vi "QEditor.vi"() -> ()   [LabVIEW 2018]
uses:
  QBuilder Files/Actions_arr.ctl
  QBuilder Files/Action.ctl
  QBuilder Files/Parameters.ctl
panel:
  in  "Tab Control":enum32{"Main", "Stored Variables", "Basher"}(tab)
  in  "Actions":T1=[{"Toggle"=TRUE, "Open parameter editor"=FALSE, "Open MacroEditor"=FALSE, "Macro path"=path "", "Duration (s)"=0.001, "Parameters"=[{"Status"="ADC", "Name"="mode (0,1,2)", "Value"=0.0, "Changed"=FALSE}, {"Status"="Camera", "Name"="state (0,1)", "Value"=0.0, "Changed"=FALSE}, {"Status"="Slave", "Name"="state (0,1)", "Value"=0.0, "Changed"=FALSE}, {"Status"="Wait", "Name"="inbit (0...7)", "Value"=0.0, "Changed"=FALSE}, {"Status"="e-", "Name"="burn time (s)", "Value"=0.0, "Changed"=FALSE}, {"Status"="e-", "Name"="filament (A)", "Value"=0.0, "Changed"=FALSE}, {"Status"="e-", "Name"="enable (0,1)", "Value"=0.0, "Changed"=FALSE}, {"Status"="RW", "Name"="mode (0-13)", "Value"=0.0, "Changed"=FALSE}, {"Status"="RW", "Name"="f_start (Hz)", "Value"=0.0, "Changed"=FALSE}, {"Status"="RW", "Name"="f_stop (Hz)", "Value"=0.0, "Changed"=FALSE}, {"Status"="RW", "Name"="amplitude (V)", "Value"=0.0, "Changed"=FALSE}, {"Status"="RW", "Name"="phase dif (deg)", "Value"=0.0, "Changed"=FALSE}, {"Status"="RW", "Name"="sweep time (s)", "Value"=0.0, "Changed"=FALSE}, {"Status"="HVpuls1", "Name"="polarity (0=n)", "Value"=0.0, "Changed"=FALSE}, {"Status"="HVpuls1", "Name"="enable (0,1)", "Value"=0.0, "Changed"=FALSE}, {"Status"="HVpuls1", "Name"="amplitude (V)", "Value"=0.0, "Changed"=FALSE}, {"Status"="HVptime", "Name"="Mush on (0,1)", "Value"=0.0, "Changed"=FALSE}, {"Status"="HVptime", "Name"="Posi on (0,1)", "Value"=0.0, "Changed"=FALSE}, {"Status"="HVptime", "Name"="Cusp on (0,1)", "Value"=0.0, "Changed"=FALSE}, {"Status"="HVptime", "Name"="Posi width (s)", "Value"=0.0, "Changed"=FALSE}, {"Status"="HVptime", "Name"="Cusp delay (s)", "Value"=0.0, "Changed"=FALSE}, {"Status"="HVptime", "Name"="Cusp width (s)", "Value"=0.0, "Changed"=FALSE}, {"Status"="Dcoils", "Name"="Higaki A  (A)", "Value"=0.0, "Changed"=FALSE}, {"Status"="Dcoils", "Name"="Higaki B,C (A)", "Value"=0.0, "Changed"=FALSE}, {"Status"="Horn", "Name"="Klaxon (0,1)", "Value"=0.0, "Changed"=FALSE}, {"Status"="AMT", "Name"="posAMT (0,1)", "Value"=0.0, "Changed"=FALSE}, {"Status"="Scoop", "Name"="Acquisitions", "Value"=0.0, "Changed"=FALSE}, {"Status"="MCP", "Name"="front bias (V)", "Value"=0.0, "Changed"=FALSE}, {"Status"="MCP", "Name"="back bias (V)", "Value"=0.0, "Changed"=FALSE}, {"Status"="MCP", "Name"="phos bias (V)", "Value"=0.0, "Changed"=FALSE}, {"Status"="FI", "Name"="US bias (V)", "Value"=0.0, "Changed"=FALSE}, {"Status"="FI", "Name"="DS bias (V)", "Value"=0.0, "Changed"=FALSE}], "Comment"="", "Reps"=10}, {"Toggle"=FALSE, "Open parameter editor"=FALSE, "Open MacroEditor"=FALSE, "Macro path"=path "C:/CuspControl/Cusp/1_Macros/Antiprotons/Reservoir/v102/scoopDS__000.mac", "Duration (s)"=0.094, "Parameters"=[{"Status"="ADC", "Name"="mode (0,1,2)", "Value"=0.0, "Changed"=FALSE}, {"Status"="Camera", "Name"="state (0,1)", "Value"=0.0, "Changed"=FALSE}, {"Status"="Slave", "Name"="state (0,1)", "Value"=0.0, "Changed"=FALSE}, {"Status"="Wait", "Name"="inbit (0...7)", "Value"=0.0, "Changed"=FALSE}, {"Status"="e-", "Name"="burn time (s)", "Value"=0.0, "Changed"=FALSE}, {"Status"="e-", "Name"="filament (A)", "Value"=0.0, "Changed"=FALSE}, {"Status"="e-", "Name"="enable (0,1)", "Value"=0.0, "Changed"=FALSE}, {"Status"="RW", "Name"="mode (0-13)", "Value"=0.0, "Changed"=FALSE}, {"Status"="RW", "Name"="f_start (Hz)", "Value"=0.0, "Changed"=FALSE}, {"Status"="RW", "Name"="f_stop (Hz)", "Value"=0.0, "Changed"=FALSE}, {"Status"="RW", "Name"="amplitude (V)", "Value"=0.0, "Changed"=FALSE}, {"Status"="RW", "Name"="phase dif (deg)", "Value"=0.0, "Changed"=FALSE}, {"Status"="RW", "Name"="sweep time (s)", "Value"=0.0, "Changed"=FALSE}, {"Status"="HVpuls1", "Name"="polarity (0=n)", "Value"=0.0, "Changed"=FALSE}, {"Status"="HVpuls1", "Name"="enable (0,1)", "Value"=0.0, "Changed"=FALSE}, {"Status"="HVpuls1", "Name"="amplitude (V)", "Value"=0.0, "Changed"=FALSE}, {"Status"="HVptime", "Name"="Mush on (0,1)", "Value"=0.0, "Changed"=FALSE}, {"Status"="HVptime", "Name"="Posi on (0,1)", "Value"=0.0, "Changed"=FALSE}, {"Status"="HVptime", "Name"="Cusp on (0,1)", "Value"=0.0, "Changed"=FALSE}, {"Status"="HVptime", "Name"="Posi width (s)", "Value"=0.0, "Changed"=FALSE}, {"Status"="HVptime", "Name"="Cusp delay (s)", "Value"=0.0, "Changed"=FALSE}, {"Status"="HVptime", "Name"="Cusp width (s)", "Value"=0.0, "Changed"=FALSE}, {"Status"="Dcoils", "Name"="Higaki A  (A)", "Value"=0.0, "Changed"=FALSE}, {"Status"="Dcoils", "Name"="Higaki B,C (A)", "Value"=0.0, "Changed"=FALSE}, {"Status"="Horn", "Name"="Klaxon (0,1)", "Value"=0.0, "Changed"=FALSE}, {"Status"="AMT", "Name"="posAMT (0,1)", "Value"=0.0, "Changed"=FALSE}, {"Status"="Scoop", "Name"="Acquisitions", "Value"=0.0, "Changed"=FALSE}, {"Status"="MCP", "Name"="front bias (V)", "Value"=0.0, "Changed"=FALSE}, {"Status"="MCP", "Name"="back bias (V)", "Value"=0.0, "Changed"=FALSE}, {"Status"="MCP", "Name"="phos bias (V)", "Value"=0.0, "Changed"=FALSE}, {"Status"="FI", "Name"="US bias (V)", "Value"=0.0, "Changed"=FALSE}, {"Status"="FI", "Name"="DS bias (V)", "Value"=0.0, "Changed"=FALSE}], "Comment"="downstream dump\nno ekick", "Reps"=10}, {"Toggle"=FALSE, "Open parameter editor"=FALSE, "Open MacroEditor"=FALSE, "Macro path"=path "C:/CuspControl/Cusp/1_Macros/Antiprotons/Reservoir/v102/scoopDS__001.mac", "Duration (s)"=0.094, "Parameters"=[{"Status"="ADC", "Name"="mode (0,1,2)", "Value"=0.0, "Changed"=FALSE}, {"Status"="Camera", "Name"="state (0,1)", "Value"=0.0, "Changed"=FALSE}, {"Status"="Slave", "Name"="state (0,1)", "Value"=0.0, "Changed"=FALSE}, {"Status"="Wait", "Name"="inbit (0...7)", "Value"=0.0, "Changed"=FALSE}, {"Status"="e-", "Name"="burn time (s)", "Value"=0.0, "Changed"=FALSE}, {"Status"="e-", "Name"="filament (A)", "Value"=0.0, "Changed"=FALSE}, {"Status"="e-", "Name"="enable (0,1)", "Value"=0.0, "Changed"=FALSE}, {"Status"="RW", "Name"="mode (0-13)", "Value"=0.0, "Changed"=FALSE}, {"Status"="RW", "Name"="f_start (Hz)", "Value"=0.0, "Changed"=FALSE}, {"Status"="RW", "Name"="f_stop (Hz)", "Value"=0.0, "Changed"=FALSE}, {"Status"="RW", "Name"="amplitude (V)", "Value"=0.0, "Changed"=FALSE}, {"Status"="RW", "Name"="phase dif (deg)", "Value"=0.0, "Changed"=FALSE}, {"Status"="RW", "Name"="sweep time (s)", "Value"=0.0, "Changed"=FALSE}, {"Status"="HVpuls1", "Name"="polarity (0=n)", "Value"=0.0, "Changed"=FALSE}, {"Status"="HVpuls1", "Name"="enable (0,1)", "Value"=0.0, "Changed"=FALSE}, {"Status"="HVpuls1", "Name"="amplitude (V)", "Value"=0.0, "Changed"=FALSE}, {"Status"="HVptime", "Name"="Mush on (0,1)", "Value"=0.0, "Changed"=FALSE}, {"Status"="HVptime", "Name"="Posi on (0,1)", "Value"=0.0, "Changed"=FALSE}, {"Status"="HVptime", "Name"="Cusp on (0,1)", "Value"=0.0, "Changed"=FALSE}, {"Status"="HVptime", "Name"="Posi width (s)", "Value"=0.0, "Changed"=FALSE}, {"Status"="HVptime", "Name"="Cusp delay (s)", "Value"=0.0, "Changed"=FALSE}, {"Status"="HVptime", "Name"="Cusp width (s)", "Value"=0.0, "Changed"=FALSE}, {"Status"="Dcoils", "Name"="Higaki A  (A)", "Value"=0.0, "Changed"=FALSE}, {"Status"="Dcoils", "Name"="Higaki B,C (A)", "Value"=0.0, "Changed"=FALSE}, {"Status"="Horn", "Name"="Klaxon (0,1)", "Value"=0.0, "Changed"=FALSE}, {"Status"="AMT", "Name"="posAMT (0,1)", "Value"=0.0, "Changed"=FALSE}, {"Status"="Scoop", "Name"="Acquisitions", "Value"=0.0, "Changed"=FALSE}, {"Status"="MCP", "Name"="front bias (V)", "Value"=0.0, "Changed"=FALSE}, {"Status"="MCP", "Name"="back bias (V)", "Value"=0.0, "Changed"=FALSE}, {"Status"="MCP", "Name"="phos bias (V)", "Value"=0.0, "Changed"=FALSE}, {"Status"="FI", "Name"="US bias (V)", "Value"=0.0, "Changed"=FALSE}, {"Status"="FI", "Name"="DS bias (V)", "Value"=0.0, "Changed"=FALSE}], "Comment"="downstream dump\nno ekick", "Reps"=10}, {"Toggle"=FALSE, "Open parameter editor"=FALSE, "Open MacroEditor"=FALSE, "Macro path"=path "C:/CuspControl/Cusp/1_Macros/Antiprotons/Reservoir/v102/scoopDS__002.mac", "Duration (s)"=0.094, "Parameters"=[{"Status"="ADC", "Name"="mode (0,1,2)", "Value"=0.0, "Changed"=FALSE}, {"Status"="Camera", "Name"="state (0,1)", "Value"=0.0, "Changed"=FALSE}, {"Status"="Slave", "Name"="state (0,1)", "Value"=0.0, "Changed"=FALSE}, {"Status"="Wait", "Name"="inbit (0...7)", "Value"=0.0, "Changed"=FALSE}, {"Status"="e-", "Name"="burn time (s)", "Value"=0.0, "Changed"=FALSE}, {"Status"="e-", "Name"="filament (A)", "Value"=0.0, "Changed"=FALSE}, {"Status"="e-", "Name"="enable (0,1)", "Value"=0.0, "Changed"=FALSE}, {"Status"="RW", "Name"="mode (0-13)", "Value"=0.0, "Changed"=FALSE}, {"Status"="RW", "Name"="f_start (Hz)", "Value"=0.0, "Changed"=FALSE}, {"Status"="RW", "Name"="f_stop (Hz)", "Value"=0.0, "Changed"=FALSE}, {"Status"="RW", "Name"="amplitude (V)", "Value"=0.0, "Changed"=FALSE}, {"Status"="RW", "Name"="phase dif (deg)", "Value"=0.0, "Changed"=FALSE}, {"Status"="RW", "Name"="sweep time (s)", "Value"=0.0, "Changed"=FALSE}, {"Status"="HVpuls1", "Name"="polarity (0=n)", "Value"=0.0, "Changed"=FALSE}, {"Status"="HVpuls1", "Name"="enable (0,1)", "Value"=0.0, "Changed"=FALSE}, {"Status"="HVpuls1", "Name"="amplitude (V)", "Value"=0.0, "Changed"=FALSE}, {"Status"="HVptime", "Name"="Mush on (0,1)", "Value"=0.0, "Changed"=FALSE}, {"Status"="HVptime", "Name"="Posi on (0,1)", "Value"=0.0, "Changed"=FALSE}, {"Status"="HVptime", "Name"="Cusp on (0,1)", "Value"=0.0, "Changed"=FALSE}, {"Status"="HVptime", "Name"="Posi width (s)", "Value"=0.0, "Changed"=FALSE}, {"Status"="HVptime", "Name"="Cusp delay (s)", "Value"=0.0, "Changed"=FALSE}, {"Status"="HVptime", "Name"="Cusp width (s)", "Value"=0.0, "Changed"=FALSE}, {"Status"="Dcoils", "Name"="Higaki A  (A)", "Value"=0.0, "Changed"=FALSE}, {"Status"="Dcoils", "Name"="Higaki B,C (A)", "Value"=0.0, "Changed"=FALSE}, {"Status"="Horn", "Name"="Klaxon (0,1)", "Value"=0.0, "Changed"=FALSE}, {"Status"="AMT", "Name"="posAMT (0,1)", "Value"=0.0, "Changed"=FALSE}, {"Status"="Scoop", "Name"="Acquisitions", "Value"=0.0, "Changed"=FALSE}, {"Status"="MCP", "Name"="front bias (V)", "Value"=0.0, "Changed"=FALSE}, {"Status"="MCP", "Name"="back bias (V)", "Value"=0.0, "Changed"=FALSE}, {"Status"="MCP", "Name"="phos bias (V)", "Value"=0.0, "Changed"=FALSE}, {"Status"="FI", "Name"="US bias (V)", "Value"=0.0, "Changed"=FALSE}, {"Status"="FI", "Name"="DS bias (V)", "Value"=0.0, "Changed"=FALSE}], "Comment"="downstream dump\nno ekick", "Reps"=10}, {"Toggle"=FALSE, "Open parameter editor"=FALSE, "Open MacroEditor"=FALSE, "Macro path"=path "C:/CuspControl/Cusp/1_Macros/Antiprotons/Reservoir/v102/scoopDS__003.mac", "Duration (s)"=0.094, "Parameters"=[{"Status"="ADC", "Name"="mode (0,1,2)", "Value"=0.0, "Changed"=FALSE}, {"Status"="Camera", "Name"="state (0,1)", "Value"=0.0, "Changed"=FALSE}, {"Status"="Slave", "Name"="state (0,1)", "Value"=0.0, "Changed"=FALSE}, {"Status"="Wait", "Name"="inbit (0...7)", "Value"=0.0, "Changed"=FALSE}, {"Status"="e-", "Name"="burn time (s)", "Value"=0.0, "Changed"=FALSE}, {"Status"="e-", "Name"="filament (A)", "Value"=0.0, "Changed"=FALSE}, {"Status"="e-", "Name"="enable (0,1)", "Value"=0.0, "Changed"=FALSE}, {"Status"="RW", "Name"="mode (0-13)", "Value"=0.0, "Changed"=FALSE}, {"Status"="RW", "Name"="f_start (Hz)", "Value"=0.0, "Changed"=FALSE}, {"Status"="RW", "Name"="f_stop (Hz)", "Value"=0.0, "Changed"=FALSE}, {"Status"="RW", "Name"="amplitude (V)", "Value"=0.0, "Changed"=FALSE}, {"Status"="RW", "Name"="phase dif (deg)", "Value"=0.0, "Changed"=FALSE}, {"Status"="RW", "Name"="sweep time (s)", "Value"=0.0, "Changed"=FALSE}, {"Status"="HVpuls1", "Name"="polarity (0=n)", "Value"=0.0, "Changed"=FALSE}, {"Status"="HVpuls1", "Name"="enable (0,1)", "Value"=0.0, "Changed"=FALSE}, {"Status"="HVpuls1", "Name"="amplitude (V)", "Value"=0.0, "Changed"=FALSE}, {"Status"="HVptime", "Name"="Mush on (0,1)", "Value"=0.0, "Changed"=FALSE}, {"Status"="HVptime", "Name"="Posi on (0,1)", "Value"=0.0, "Changed"=FALSE}, {"Status"="HVptime", "Name"="Cusp on (0,1)", "Value"=0.0, "Changed"=FALSE}, {"Status"="HVptime", "Name"="Posi width (s)", "Value"=0.0, "Changed"=FALSE}, {"Status"="HVptime", "Name"="Cusp delay (s)", "Value"=0.0, "Changed"=FALSE}, {"Status"="HVptime", "Name"="Cusp width (s)", "Value"=0.0, "Changed"=FALSE}, {"Status"="Dcoils", "Name"="Higaki A  (A)", "Value"=0.0, "Changed"=FALSE}, {"Status"="Dcoils", "Name"="Higaki B,C (A)", "Value"=0.0, "Changed"=FALSE}, {"Status"="Horn", "Name"="Klaxon (0,1)", "Value"=0.0, "Changed"=FALSE}, {"Status"="AMT", "Name"="posAMT (0,1)", "Value"=0.0, "Changed"=FALSE}, {"Status"="Scoop", "Name"="Acquisitions", "Value"=0.0, "Changed"=FALSE}, {"Status"="MCP", "Name"="front bias (V)", "Value"=0.0, "Changed"=FALSE}, {"Status"="MCP", "Name"="back bias (V)", "Value"=0.0, "Changed"=FALSE}, {"Status"="MCP", "Name"="phos bias (V)", "Value"=0.0, "Changed"=FALSE}, {"Status"="FI", "Name"="US bias (V)", "Value"=0.0, "Changed"=FALSE}, {"Status"="FI", "Name"="DS bias (V)", "Value"=0.0, "Changed"=FALSE}], "Comment"="downstream dump\nno ekick", "Reps"=10}, {"Toggle"=FALSE, "Open parameter editor"=FALSE, "Open MacroEditor"=FALSE, "Macro path"=path "C:/CuspControl/Cusp/1_Macros/Antiprotons/Reservoir/v102/scoopDS__004.mac", "Duration (s)"=0.094, "Parameters"=[{"Status"="ADC", "Name"="mode (0,1,2)", "Value"=0.0, "Changed"=FALSE}, {"Status"="Camera", "Name"="state (0,1)", "Value"=0.0, "Changed"=FALSE}, {"Status"="Slave", "Name"="state (0,1)", "Value"=0.0, "Changed"=FALSE}, {"Status"="Wait", "Name"="inbit (0...7)", "Value"=0.0, "Changed"=FALSE}, {"Status"="e-", "Name"="burn time (s)", "Value"=0.0, "Changed"=FALSE}, {"Status"="e-", "Name"="filament (A)", "Value"=0.0, "Changed"=FALSE}, {"Status"="e-", "Name"="enable (0,1)", "Value"=0.0, "Changed"=FALSE}, {"Status"="RW", "Name"="mode (0-13)", "Value"=0.0, "Changed"=FALSE}, {"Status"="RW", "Name"="f_start (Hz)", "Value"=0.0, "Changed"=FALSE}, {"Status"="RW", "Name"="f_stop (Hz)", "Value"=0.0, "Changed"=FALSE}, {"Status"="RW", "Name"="amplitude (V)", "Value"=0.0, "Changed"=FALSE}, {"Status"="RW", "Name"="phase dif (deg)", "Value"=0.0, "Changed"=FALSE}, {"Status"="RW", "Name"="sweep time (s)", "Value"=0.0, "Changed"=FALSE}, {"Status"="HVpuls1", "Name"="polarity (0=n)", "Value"=0.0, "Changed"=FALSE}, {"Status"="HVpuls1", "Name"="enable (0,1)", "Value"=0.0, "Changed"=FALSE}, {"Status"="HVpuls1", "Name"="amplitude (V)", "Value"=0.0, "Changed"=FALSE}, {"Status"="HVptime", "Name"="Mush on (0,1)", "Value"=0.0, "Changed"=FALSE}, {"Status"="HVptime", "Name"="Posi on (0,1)", "Value"=0.0, "Changed"=FALSE}, {"Status"="HVptime", "Name"="Cusp on (0,1)", "Value"=0.0, "Changed"=FALSE}, {"Status"="HVptime", "Name"="Posi width (s)", "Value"=0.0, "Changed"=FALSE}, {"Status"="HVptime", "Name"="Cusp delay (s)", "Value"=0.0, "Changed"=FALSE}, {"Status"="HVptime", "Name"="Cusp width (s)", "Value"=0.0, "Changed"=FALSE}, {"Status"="Dcoils", "Name"="Higaki A  (A)", "Value"=0.0, "Changed"=FALSE}, {"Status"="Dcoils", "Name"="Higaki B,C (A)", "Value"=0.0, "Changed"=FALSE}, {"Status"="Horn", "Name"="Klaxon (0,1)", "Value"=0.0, "Changed"=FALSE}, {"Status"="AMT", "Name"="posAMT (0,1)", "Value"=0.0, "Changed"=FALSE}, {"Status"="Scoop", "Name"="Acquisitions", "Value"=0.0, "Changed"=FALSE}, {"Status"="MCP", "Name"="front bias (V)", "Value"=0.0, "Changed"=FALSE}, {"Status"="MCP", "Name"="back bias (V)", "Value"=0.0, "Changed"=FALSE}, {"Status"="MCP", "Name"="phos bias (V)", "Value"=0.0, "Changed"=FALSE}, {"Status"="FI", "Name"="US bias (V)", "Value"=0.0, "Changed"=FALSE}, {"Status"="FI", "Name"="DS bias (V)", "Value"=0.0, "Changed"=FALSE}], "Comment"="downstream dump\nno ekick", "Reps"=10}, {"Toggle"=FALSE, "Open parameter editor"=FALSE, "Open MacroEditor"=FALSE, "Macro path"=path "C:/CuspControl/Cusp/1_Macros/Antiprotons/Reservoir/v102/scoopDS__005.mac", "Duration (s)"=0.094, "Parameters"=[{"Status"="ADC", "Name"="mode (0,1,2)", "Value"=0.0, "Changed"=FALSE}, {"Status"="Camera", "Name"="state (0,1)", "Value"=0.0, "Changed"=FALSE}, {"Status"="Slave", "Name"="state (0,1)", "Value"=0.0, "Changed"=FALSE}, {"Status"="Wait", "Name"="inbit (0...7)", "Value"=0.0, "Changed"=FALSE}, {"Status"="e-", "Name"="burn time (s)", "Value"=0.0, "Changed"=FALSE}, {"Status"="e-", "Name"="filament (A)", "Value"=0.0, "Changed"=FALSE}, {"Status"="e-", "Name"="enable (0,1)", "Value"=0.0, "Changed"=FALSE}, {"Status"="RW", "Name"="mode (0-13)", "Value"=0.0, "Changed"=FALSE}, {"Status"="RW", "Name"="f_start (Hz)", "Value"=0.0, "Changed"=FALSE}, {"Status"="RW", "Name"="f_stop (Hz)", "Value"=0.0, "Changed"=FALSE}, {"Status"="RW", "Name"="amplitude (V)", "Value"=0.0, "Changed"=FALSE}, {"Status"="RW", "Name"="phase dif (deg)", "Value"=0.0, "Changed"=FALSE}, {"Status"="RW", "Name"="sweep time (s)", "Value"=0.0, "Changed"=FALSE}, {"Status"="HVpuls1", "Name"="polarity (0=n)", "Value"=0.0, "Changed"=FALSE}, {"Status"="HVpuls1", "Name"="enable (0,1)", "Value"=0.0, "Changed"=FALSE}, {"Status"="HVpuls1", "Name"="amplitude (V)", "Value"=0.0, "Changed"=FALSE}, {"Status"="HVptime", "Name"="Mush on (0,1)", "Value"=0.0, "Changed"=FALSE}, {"Status"="HVptime", "Name"="Posi on (0,1)", "Value"=0.0, "Changed"=FALSE}, {"Status"="HVptime", "Name"="Cusp on (0,1)", "Value"=0.0, "Changed"=FALSE}, {"Status"="HVptime", "Name"="Posi width (s)", "Value"=0.0, "Changed"=FALSE}, {"Status"="HVptime", "Name"="Cusp delay (s)", "Value"=0.0, "Changed"=FALSE}, {"Status"="HVptime", "Name"="Cusp width (s)", "Value"=0.0, "Changed"=FALSE}, {"Status"="Dcoils", "Name"="Higaki A  (A)", "Value"=0.0, "Changed"=FALSE}, {"Status"="Dcoils", "Name"="Higaki B,C (A)", "Value"=0.0, "Changed"=FALSE}, {"Status"="Horn", "Name"="Klaxon (0,1)", "Value"=0.0, "Changed"=FALSE}, {"Status"="AMT", "Name"="posAMT (0,1)", "Value"=0.0, "Changed"=FALSE}, {"Status"="Scoop", "Name"="Acquisitions", "Value"=0.0, "Changed"=FALSE}, {"Status"="MCP", "Name"="front bias (V)", "Value"=0.0, "Changed"=FALSE}, {"Status"="MCP", "Name"="back bias (V)", "Value"=0.0, "Changed"=FALSE}, {"Status"="MCP", "Name"="phos bias (V)", "Value"=0.0, "Changed"=FALSE}, {"Status"="FI", "Name"="US bias (V)", "Value"=0.0, "Changed"=FALSE}, {"Status"="FI", "Name"="DS bias (V)", "Value"=0.0, "Changed"=FALSE}], "Comment"="downstream dump\nno ekick", "Reps"=10}, {"Toggle"=FALSE, "Open parameter editor"=FALSE, "Open MacroEditor"=FALSE, "Macro path"=path "C:/CuspControl/Cusp/1_Macros/Antiprotons/Reservoir/v102/scoopDS__006.mac", "Duration (s)"=0.094, "Parameters"=[{"Status"="ADC", "Name"="mode (0,1,2)", "Value"=0.0, "Changed"=FALSE}, {"Status"="Camera", "Name"="state (0,1)", "Value"=0.0, "Changed"=FALSE}, {"Status"="Slave", "Name"="state (0,1)", "Value"=0.0, "Changed"=FALSE}, {"Status"="Wait", "Name"="inbit (0...7)", "Value"=0.0, "Changed"=FALSE}, {"Status"="e-", "Name"="burn time (s)", "Value"=0.0, "Changed"=FALSE}, {"Status"="e-", "Name"="filament (A)", "Value"=0.0, "Changed"=FALSE}, {"Status"="e-", "Name"="enable (0,1)", "Value"=0.0, "Changed"=FALSE}, {"Status"="RW", "Name"="mode (0-13)", "Value"=0.0, "Changed"=FALSE}, {"Status"="RW", "Name"="f_start (Hz)", "Value"=0.0, "Changed"=FALSE}, {"Status"="RW", "Name"="f_stop (Hz)", "Value"=0.0, "Changed"=FALSE}, {"Status"="RW", "Name"="amplitude (V)", "Value"=0.0, "Changed"=FALSE}, {"Status"="RW", "Name"="phase dif (deg)", "Value"=0.0, "Changed"=FALSE}, {"Status"="RW", "Name"="sweep time (s)", "Value"=0.0, "Changed"=FALSE}, {"Status"="HVpuls1", "Name"="polarity (0=n)", "Value"=0.0, "Changed"=FALSE}, {"Status"="HVpuls1", "Name"="enable (0,1)", "Value"=0.0, "Changed"=FALSE}, {"Status"="HVpuls1", "Name"="amplitude (V)", "Value"=0.0, "Changed"=FALSE}, {"Status"="HVptime", "Name"="Mush on (0,1)", "Value"=0.0, "Changed"=FALSE}, {"Status"="HVptime", "Name"="Posi on (0,1)", "Value"=0.0, "Changed"=FALSE}, {"Status"="HVptime", "Name"="Cusp on (0,1)", "Value"=0.0, "Changed"=FALSE}, {"Status"="HVptime", "Name"="Posi width (s)", "Value"=0.0, "Changed"=FALSE}, {"Status"="HVptime", "Name"="Cusp delay (s)", "Value"=0.0, "Changed"=FALSE}, {"Status"="HVptime", "Name"="Cusp width (s)", "Value"=0.0, "Changed"=FALSE}, {"Status"="Dcoils", "Name"="Higaki A  (A)", "Value"=0.0, "Changed"=FALSE}, {"Status"="Dcoils", "Name"="Higaki B,C (A)", "Value"=0.0, "Changed"=FALSE}, {"Status"="Horn", "Name"="Klaxon (0,1)", "Value"=0.0, "Changed"=FALSE}, {"Status"="AMT", "Name"="posAMT (0,1)", "Value"=0.0, "Changed"=FALSE}, {"Status"="Scoop", "Name"="Acquisitions", "Value"=0.0, "Changed"=FALSE}, {"Status"="MCP", "Name"="front bias (V)", "Value"=0.0, "Changed"=FALSE}, {"Status"="MCP", "Name"="back bias (V)", "Value"=0.0, "Changed"=FALSE}, {"Status"="MCP", "Name"="phos bias (V)", "Value"=0.0, "Changed"=FALSE}, {"Status"="FI", "Name"="US bias (V)", "Value"=0.0, "Changed"=FALSE}, {"Status"="FI", "Name"="DS bias (V)", "Value"=0.0, "Changed"=FALSE}], "Comment"="downstream dump\nno ekick", "Reps"=10}, {"Toggle"=FALSE, "Open parameter editor"=FALSE, "Open MacroEditor"=FALSE, "Macro path"=path "C:/CuspControl/Cusp/1_Macros/Antiprotons/Reservoir/v102/scoopDS__007.mac", "Duration (s)"=0.094, "Parameters"=[{"Status"="ADC", "Name"="mode (0,1,2)", "Value"=0.0, "Changed"=FALSE}, {"Status"="Camera", "Name"="state (0,1)", "Value"=0.0, "Changed"=FALSE}, {"Status"="Slave", "Name"="state (0,1)", "Value"=0.0, "Changed"=FALSE}, {"Status"="Wait", "Name"="inbit (0...7)", "Value"=0.0, "Changed"=FALSE}, {"Status"="e-", "Name"="burn time (s)", "Value"=0.0, "Changed"=FALSE}, {"Status"="e-", "Name"="filament (A)", "Value"=0.0, "Changed"=FALSE}, {"Status"="e-", "Name"="enable (0,1)", "Value"=0.0, "Changed"=FALSE}, {"Status"="RW", "Name"="mode (0-13)", "Value"=0.0, "Changed"=FALSE}, {"Status"="RW", "Name"="f_start (Hz)", "Value"=0.0, "Changed"=FALSE}, {"Status"="RW", "Name"="f_stop (Hz)", "Value"=0.0, "Changed"=FALSE}, {"Status"="RW", "Name"="amplitude (V)", "Value"=0.0, "Changed"=FALSE}, {"Status"="RW", "Name"="phase dif (deg)", "Value"=0.0, "Changed"=FALSE}, {"Status"="RW", "Name"="sweep time (s)", "Value"=0.0, "Changed"=FALSE}, {"Status"="HVpuls1", "Name"="polarity (0=n)", "Value"=0.0, "Changed"=FALSE}, {"Status"="HVpuls1", "Name"="enable (0,1)", "Value"=0.0, "Changed"=FALSE}, {"Status"="HVpuls1", "Name"="amplitude (V)", "Value"=0.0, "Changed"=FALSE}, {"Status"="HVptime", "Name"="Mush on (0,1)", "Value"=0.0, "Changed"=FALSE}, {"Status"="HVptime", "Name"="Posi on (0,1)", "Value"=0.0, "Changed"=FALSE}, {"Status"="HVptime", "Name"="Cusp on (0,1)", "Value"=0.0, "Changed"=FALSE}, {"Status"="HVptime", "Name"="Posi width (s)", "Value"=0.0, "Changed"=FALSE}, {"Status"="HVptime", "Name"="Cusp delay (s)", "Value"=0.0, "Changed"=FALSE}, {"Status"="HVptime", "Name"="Cusp width (s)", "Value"=0.0, "Changed"=FALSE}, {"Status"="Dcoils", "Name"="Higaki A  (A)", "Value"=0.0, "Changed"=FALSE}, {"Status"="Dcoils", "Name"="Higaki B,C (A)", "Value"=0.0, "Changed"=FALSE}, {"Status"="Horn", "Name"="Klaxon (0,1)", "Value"=0.0, "Changed"=FALSE}, {"Status"="AMT", "Name"="posAMT (0,1)", "Value"=0.0, "Changed"=FALSE}, {"Status"="Scoop", "Name"="Acquisitions", "Value"=0.0, "Changed"=FALSE}, {"Status"="MCP", "Name"="front bias (V)", "Value"=0.0, "Changed"=FALSE}, {"Status"="MCP", "Name"="back bias (V)", "Value"=0.0, "Changed"=FALSE}, {"Status"="MCP", "Name"="phos bias (V)", "Value"=0.0, "Changed"=FALSE}, {"Status"="FI", "Name"="US bias (V)", "Value"=0.0, "Changed"=FALSE}, {"Status"="FI", "Name"="DS bias (V)", "Value"=0.0, "Changed"=FALSE}], "Comment"="downstream dump\nno ekick", "Reps"=10}, {"Toggle"=FALSE, "Open parameter editor"=FALSE, "Open MacroEditor"=FALSE, "Macro path"=path "C:/CuspControl/Cusp/1_Macros/Antiprotons/Reservoir/v102/scoopDS__008.mac", "Duration (s)"=0.094, "Parameters"=[{"Status"="ADC", "Name"="mode (0,1,2)", "Value"=0.0, "Changed"=FALSE}, {"Status"="Camera", "Name"="state (0,1)", "Value"=0.0, "Changed"=FALSE}, {"Status"="Slave", "Name"="state (0,1)", "Value"=0.0, "Changed"=FALSE}, {"Status"="Wait", "Name"="inbit (0...7)", "Value"=0.0, "Changed"=FALSE}, {"Status"="e-", "Name"="burn time (s)", "Value"=0.0, "Changed"=FALSE}, {"Status"="e-", "Name"="filament (A)", "Value"=0.0, "Changed"=FALSE}, {"Status"="e-", "Name"="enable (0,1)", "Value"=0.0, "Changed"=FALSE}, {"Status"="RW", "Name"="mode (0-13)", "Value"=0.0, "Changed"=FALSE}, {"Status"="RW", "Name"="f_start (Hz)", "Value"=0.0, "Changed"=FALSE}, {"Status"="RW", "Name"="f_stop (Hz)", "Value"=0.0, "Changed"=FALSE}, {"Status"="RW", "Name"="amplitude (V)", "Value"=0.0, "Changed"=FALSE}, {"Status"="RW", "Name"="phase dif (deg)", "Value"=0.0, "Changed"=FALSE}, {"Status"="RW", "Name"="sweep time (s)", "Value"=0.0, "Changed"=FALSE}, {"Status"="HVpuls1", "Name"="polarity (0=n)", "Value"=0.0, "Changed"=FALSE}, {"Status"="HVpuls1", "Name"="enable (0,1)", "Value"=0.0, "Changed"=FALSE}, {"Status"="HVpuls1", "Name"="amplitude (V)", "Value"=0.0, "Changed"=FALSE}, {"Status"="HVptime", "Name"="Mush on (0,1)", "Value"=0.0, "Changed"=FALSE}, {"Status"="HVptime", "Name"="Posi on (0,1)", "Value"=0.0, "Changed"=FALSE}, {"Status"="HVptime", "Name"="Cusp on (0,1)", "Value"=0.0, "Changed"=FALSE}, {"Status"="HVptime", "Name"="Posi width (s)", "Value"=0.0, "Changed"=FALSE}, {"Status"="HVptime", "Name"="Cusp delay (s)", "Value"=0.0, "Changed"=FALSE}, {"Status"="HVptime", "Name"="Cusp width (s)", "Value"=0.0, "Changed"=FALSE}, {"Status"="Dcoils", "Name"="Higaki A  (A)", "Value"=0.0, "Changed"=FALSE}, {"Status"="Dcoils", "Name"="Higaki B,C (A)", "Value"=0.0, "Changed"=FALSE}, {"Status"="Horn", "Name"="Klaxon (0,1)", "Value"=0.0, "Changed"=FALSE}, {"Status"="AMT", "Name"="posAMT (0,1)", "Value"=0.0, "Changed"=FALSE}, {"Status"="Scoop", "Name"="Acquisitions", "Value"=0.0, "Changed"=FALSE}, {"Status"="MCP", "Name"="front bias (V)", "Value"=0.0, "Changed"=FALSE}, {"Status"="MCP", "Name"="back bias (V)", "Value"=0.0, "Changed"=FALSE}, {"Status"="MCP", "Name"="phos bias (V)", "Value"=0.0, "Changed"=FALSE}, {"Status"="FI", "Name"="US bias (V)", "Value"=0.0, "Changed"=FALSE}, {"Status"="FI", "Name"="DS bias (V)", "Value"=0.0, "Changed"=FALSE}], "Comment"="downstream dump\nno ekick", "Reps"=10}, {"Toggle"=FALSE, "Open parameter editor"=FALSE, "Open MacroEditor"=FALSE, "Macro path"=path "C:/CuspControl/Cusp/1_Macros/Antiprotons/Reservoir/v102/scoopDS__009.mac", "Duration (s)"=0.094, "Parameters"=[{"Status"="ADC", "Name"="mode (0,1,2)", "Value"=0.0, "Changed"=FALSE}, {"Status"="Camera", "Name"="state (0,1)", "Value"=0.0, "Changed"=FALSE}, {"Status"="Slave", "Name"="state (0,1)", "Value"=0.0, "Changed"=FALSE}, {"Status"="Wait", "Name"="inbit (0...7)", "Value"=0.0, "Changed"=FALSE}, {"Status"="e-", "Name"="burn time (s)", "Value"=0.0, "Changed"=FALSE}, {"Status"="e-", "Name"="filament (A)", "Value"=0.0, "Changed"=FALSE}, {"Status"="e-", "Name"="enable (0,1)", "Value"=0.0, "Changed"=FALSE}, {"Status"="RW", "Name"="mode (0-13)", "Value"=0.0, "Changed"=FALSE}, {"Status"="RW", "Name"="f_start (Hz)", "Value"=0.0, "Changed"=FALSE}, {"Status"="RW", "Name"="f_stop (Hz)", "Value"=0.0, "Changed"=FALSE}, {"Status"="RW", "Name"="amplitude (V)", "Value"=0.0, "Changed"=FALSE}, {"Status"="RW", "Name"="phase dif (deg)", "Value"=0.0, "Changed"=FALSE}, {"Status"="RW", "Name"="sweep time (s)", "Value"=0.0, "Changed"=FALSE}, {"Status"="HVpuls1", "Name"="polarity (0=n)", "Value"=0.0, "Changed"=FALSE}, {"Status"="HVpuls1", "Name"="enable (0,1)", "Value"=0.0, "Changed"=FALSE}, {"Status"="HVpuls1", "Name"="amplitude (V)", "Value"=0.0, "Changed"=FALSE}, {"Status"="HVptime", "Name"="Mush on (0,1)", "Value"=0.0, "Changed"=FALSE}, {"Status"="HVptime", "Name"="Posi on (0,1)", "Value"=0.0, "Changed"=FALSE}, {"Status"="HVptime", "Name"="Cusp on (0,1)", "Value"=0.0, "Changed"=FALSE}, {"Status"="HVptime", "Name"="Posi width (s)", "Value"=0.0, "Changed"=FALSE}, {"Status"="HVptime", "Name"="Cusp delay (s)", "Value"=0.0, "Changed"=FALSE}, {"Status"="HVptime", "Name"="Cusp width (s)", "Value"=0.0, "Changed"=FALSE}, {"Status"="Dcoils", "Name"="Higaki A  (A)", "Value"=0.0, "Changed"=FALSE}, {"Status"="Dcoils", "Name"="Higaki B,C (A)", "Value"=0.0, "Changed"=FALSE}, {"Status"="Horn", "Name"="Klaxon (0,1)", "Value"=0.0, "Changed"=FALSE}, {"Status"="AMT", "Name"="posAMT (0,1)", "Value"=0.0, "Changed"=FALSE}, {"Status"="Scoop", "Name"="Acquisitions", "Value"=0.0, "Changed"=FALSE}, {"Status"="MCP", "Name"="front bias (V)", "Value"=0.0, "Changed"=FALSE}, {"Status"="MCP", "Name"="back bias (V)", "Value"=0.0, "Changed"=FALSE}, {"Status"="MCP", "Name"="phos bias (V)", "Value"=0.0, "Changed"=FALSE}, {"Status"="FI", "Name"="US bias (V)", "Value"=0.0, "Changed"=FALSE}, {"Status"="FI", "Name"="DS bias (V)", "Value"=0.0, "Changed"=FALSE}], "Comment"="downstream dump\nno ekick", "Reps"=10}, {"Toggle"=FALSE, "Open parameter editor"=FALSE, "Open MacroEditor"=FALSE, "Macro path"=path "C:/CuspControl/Cusp/1_Macros/Antiprotons/Reservoir/v102/scoopDS__010.mac", "Duration (s)"=0.094, "Parameters"=[{"Status"="ADC", "Name"="mode (0,1,2)", "Value"=0.0, "Changed"=FALSE}, {"Status"="Camera", "Name"="state (0,1)", "Value"=0.0, "Changed"=FALSE}, {"Status"="Slave", "Name"="state (0,1)", "Value"=0.0, "Changed"=FALSE}, {"Status"="Wait", "Name"="inbit (0...7)", "Value"=0.0, "Changed"=FALSE}, {"Status"="e-", "Name"="burn time (s)", "Value"=0.0, "Changed"=FALSE}, {"Status"="e-", "Name"="filament (A)", "Value"=0.0, "Changed"=FALSE}, {"Status"="e-", "Name"="enable (0,1)", "Value"=0.0, "Changed"=FALSE}, {"Status"="RW", "Name"="mode (0-13)", "Value"=0.0, "Changed"=FALSE}, {"Status"="RW", "Name"="f_start (Hz)", "Value"=0.0, "Changed"=FALSE}, {"Status"="RW", "Name"="f_stop (Hz)", "Value"=0.0, "Changed"=FALSE}, {"Status"="RW", "Name"="amplitude (V)", "Value"=0.0, "Changed"=FALSE}, {"Status"="RW", "Name"="phase dif (deg)", "Value"=0.0, "Changed"=FALSE}, {"Status"="RW", "Name"="sweep time (s)", "Value"=0.0, "Changed"=FALSE}, {"Status"="HVpuls1", "Name"="polarity (0=n)", "Value"=0.0, "Changed"=FALSE}, {"Status"="HVpuls1", "Name"="enable (0,1)", "Value"=0.0, "Changed"=FALSE}, {"Status"="HVpuls1", "Name"="amplitude (V)", "Value"=0.0, "Changed"=FALSE}, {"Status"="HVptime", "Name"="Mush on (0,1)", "Value"=0.0, "Changed"=FALSE}, {"Status"="HVptime", "Name"="Posi on (0,1)", "Value"=0.0, "Changed"=FALSE}, {"Status"="HVptime", "Name"="Cusp on (0,1)", "Value"=0.0, "Changed"=FALSE}, {"Status"="HVptime", "Name"="Posi width (s)", "Value"=0.0, "Changed"=FALSE}, {"Status"="HVptime", "Name"="Cusp delay (s)", "Value"=0.0, "Changed"=FALSE}, {"Status"="HVptime", "Name"="Cusp width (s)", "Value"=0.0, "Changed"=FALSE}, {"Status"="Dcoils", "Name"="Higaki A  (A)", "Value"=0.0, "Changed"=FALSE}, {"Status"="Dcoils", "Name"="Higaki B,C (A)", "Value"=0.0, "Changed"=FALSE}, {"Status"="Horn", "Name"="Klaxon (0,1)", "Value"=0.0, "Changed"=FALSE}, {"Status"="AMT", "Name"="posAMT (0,1)", "Value"=0.0, "Changed"=FALSE}, {"Status"="Scoop", "Name"="Acquisitions", "Value"=0.0, "Changed"=FALSE}, {"Status"="MCP", "Name"="front bias (V)", "Value"=0.0, "Changed"=FALSE}, {"Status"="MCP", "Name"="back bias (V)", "Value"=0.0, "Changed"=FALSE}, {"Status"="MCP", "Name"="phos bias (V)", "Value"=0.0, "Changed"=FALSE}, {"Status"="FI", "Name"="US bias (V)", "Value"=0.0, "Changed"=FALSE}, {"Status"="FI", "Name"="DS bias (V)", "Value"=0.0, "Changed"=FALSE}], "Comment"="downstream dump\nno ekick", "Reps"=10}, {"Toggle"=FALSE, "Open parameter editor"=FALSE, "Open MacroEditor"=FALSE, "Macro path"=path "C:/CuspControl/Cusp/1_Macros/Antiprotons/Reservoir/v102/scoopDS__011.mac", "Duration (s)"=0.094, "Parameters"=[{"Status"="ADC", "Name"="mode (0,1,2)", "Value"=0.0, "Changed"=FALSE}, {"Status"="Camera", "Name"="state (0,1)", "Value"=0.0, "Changed"=FALSE}, {"Status"="Slave", "Name"="state (0,1)", "Value"=0.0, "Changed"=FALSE}, {"Status"="Wait", "Name"="inbit (0...7)", "Value"=0.0, "Changed"=FALSE}, {"Status"="e-", "Name"="burn time (s)", "Value"=0.0, "Changed"=FALSE}, {"Status"="e-", "Name"="filament (A)", "Value"=0.0, "Changed"=FALSE}, {"Status"="e-", "Name"="enable (0,1)", "Value"=0.0, "Changed"=FALSE}, {"Status"="RW", "Name"="mode (0-13)", "Value"=0.0, "Changed"=FALSE}, {"Status"="RW", "Name"="f_start (Hz)", "Value"=0.0, "Changed"=FALSE}, {"Status"="RW", "Name"="f_stop (Hz)", "Value"=0.0, "Changed"=FALSE}, {"Status"="RW", "Name"="amplitude (V)", "Value"=0.0, "Changed"=FALSE}, {"Status"="RW", "Name"="phase dif (deg)", "Value"=0.0, "Changed"=FALSE}, {"Status"="RW", "Name"="sweep time (s)", "Value"=0.0, "Changed"=FALSE}, {"Status"="HVpuls1", "Name"="polarity (0=n)", "Value"=0.0, "Changed"=FALSE}, {"Status"="HVpuls1", "Name"="enable (0,1)", "Value"=0.0, "Changed"=FALSE}, {"Status"="HVpuls1", "Name"="amplitude (V)", "Value"=0.0, "Changed"=FALSE}, {"Status"="HVptime", "Name"="Mush on (0,1)", "Value"=0.0, "Changed"=FALSE}, {"Status"="HVptime", "Name"="Posi on (0,1)", "Value"=0.0, "Changed"=FALSE}, {"Status"="HVptime", "Name"="Cusp on (0,1)", "Value"=0.0, "Changed"=FALSE}, {"Status"="HVptime", "Name"="Posi width (s)", "Value"=0.0, "Changed"=FALSE}, {"Status"="HVptime", "Name"="Cusp delay (s)", "Value"=0.0, "Changed"=FALSE}, {"Status"="HVptime", "Name"="Cusp width (s)", "Value"=0.0, "Changed"=FALSE}, {"Status"="Dcoils", "Name"="Higaki A  (A)", "Value"=0.0, "Changed"=FALSE}, {"Status"="Dcoils", "Name"="Higaki B,C (A)", "Value"=0.0, "Changed"=FALSE}, {"Status"="Horn", "Name"="Klaxon (0,1)", "Value"=0.0, "Changed"=FALSE}, {"Status"="AMT", "Name"="posAMT (0,1)", "Value"=0.0, "Changed"=FALSE}, {"Status"="Scoop", "Name"="Acquisitions", "Value"=0.0, "Changed"=FALSE}, {"Status"="MCP", "Name"="front bias (V)", "Value"=0.0, "Changed"=FALSE}, {"Status"="MCP", "Name"="back bias (V)", "Value"=0.0, "Changed"=FALSE}, {"Status"="MCP", "Name"="phos bias (V)", "Value"=0.0, "Changed"=FALSE}, {"Status"="FI", "Name"="US bias (V)", "Value"=0.0, "Changed"=FALSE}, {"Status"="FI", "Name"="DS bias (V)", "Value"=0.0, "Changed"=FALSE}], "Comment"="downstream dump\nno ekick", "Reps"=10}, {"Toggle"=FALSE, "Open parameter editor"=FALSE, "Open MacroEditor"=FALSE, "Macro path"=path "C:/CuspControl/Cusp/1_Macros/Antiprotons/Reservoir/v102/scoopDS__012.mac", "Duration (s)"=0.094, "Parameters"=[{"Status"="ADC", "Name"="mode (0,1,2)", "Value"=0.0, "Changed"=FALSE}, {"Status"="Camera", "Name"="state (0,1)", "Value"=0.0, "Changed"=FALSE}, {"Status"="Slave", "Name"="state (0,1)", "Value"=0.0, "Changed"=FALSE}, {"Status"="Wait", "Name"="inbit (0...7)", "Value"=0.0, "Changed"=FALSE}, {"Status"="e-", "Name"="burn time (s)", "Value"=0.0, "Changed"=FALSE}, {"Status"="e-", "Name"="filament (A)", "Value"=0.0, "Changed"=FALSE}, {"Status"="e-", "Name"="enable (0,1)", "Value"=0.0, "Changed"=FALSE}, {"Status"="RW", "Name"="mode (0-13)", "Value"=0.0, "Changed"=FALSE}, {"Status"="RW", "Name"="f_start (Hz)", "Value"=0.0, "Changed"=FALSE}, {"Status"="RW", "Name"="f_stop (Hz)", "Value"=0.0, "Changed"=FALSE}, {"Status"="RW", "Name"="amplitude (V)", "Value"=0.0, "Changed"=FALSE}, {"Status"="RW", "Name"="phase dif (deg)", "Value"=0.0, "Changed"=FALSE}, {"Status"="RW", "Name"="sweep time (s)", "Value"=0.0, "Changed"=FALSE}, {"Status"="HVpuls1", "Name"="polarity (0=n)", "Value"=0.0, "Changed"=FALSE}, {"Status"="HVpuls1", "Name"="enable (0,1)", "Value"=0.0, "Changed"=FALSE}, {"Status"="HVpuls1", "Name"="amplitude (V)", "Value"=0.0, "Changed"=FALSE}, {"Status"="HVptime", "Name"="Mush on (0,1)", "Value"=0.0, "Changed"=FALSE}, {"Status"="HVptime", "Name"="Posi on (0,1)", "Value"=0.0, "Changed"=FALSE}, {"Status"="HVptime", "Name"="Cusp on (0,1)", "Value"=0.0, "Changed"=FALSE}, {"Status"="HVptime", "Name"="Posi width (s)", "Value"=0.0, "Changed"=FALSE}, {"Status"="HVptime", "Name"="Cusp delay (s)", "Value"=0.0, "Changed"=FALSE}, {"Status"="HVptime", "Name"="Cusp width (s)", "Value"=0.0, "Changed"=FALSE}, {"Status"="Dcoils", "Name"="Higaki A  (A)", "Value"=0.0, "Changed"=FALSE}, {"Status"="Dcoils", "Name"="Higaki B,C (A)", "Value"=0.0, "Changed"=FALSE}, {"Status"="Horn", "Name"="Klaxon (0,1)", "Value"=0.0, "Changed"=FALSE}, {"Status"="AMT", "Name"="posAMT (0,1)", "Value"=0.0, "Changed"=FALSE}, {"Status"="Scoop", "Name"="Acquisitions", "Value"=0.0, "Changed"=FALSE}, {"Status"="MCP", "Name"="front bias (V)", "Value"=0.0, "Changed"=FALSE}, {"Status"="MCP", "Name"="back bias (V)", "Value"=0.0, "Changed"=FALSE}, {"Status"="MCP", "Name"="phos bias (V)", "Value"=0.0, "Changed"=FALSE}, {"Status"="FI", "Name"="US bias (V)", "Value"=0.0, "Changed"=FALSE}, {"Status"="FI", "Name"="DS bias (V)", "Value"=0.0, "Changed"=FALSE}], "Comment"="downstream dump\nno ekick", "Reps"=10}, {"Toggle"=FALSE, "Open parameter editor"=FALSE, "Open MacroEditor"=FALSE, "Macro path"=path "C:/CuspControl/Cusp/1_Macros/Antiprotons/Reservoir/v102/scoopDS__013.mac", "Duration (s)"=0.094, "Parameters"=[{"Status"="ADC", "Name"="mode (0,1,2)", "Value"=0.0, "Changed"=FALSE}, {"Status"="Camera", "Name"="state (0,1)", "Value"=0.0, "Changed"=FALSE}, {"Status"="Slave", "Name"="state (0,1)", "Value"=0.0, "Changed"=FALSE}, {"Status"="Wait", "Name"="inbit (0...7)", "Value"=0.0, "Changed"=FALSE}, {"Status"="e-", "Name"="burn time (s)", "Value"=0.0, "Changed"=FALSE}, {"Status"="e-", "Name"="filament (A)", "Value"=0.0, "Changed"=FALSE}, {"Status"="e-", "Name"="enable (0,1)", "Value"=0.0, "Changed"=FALSE}, {"Status"="RW", "Name"="mode (0-13)", "Value"=0.0, "Changed"=FALSE}, {"Status"="RW", "Name"="f_start (Hz)", "Value"=0.0, "Changed"=FALSE}, {"Status"="RW", "Name"="f_stop (Hz)", "Value"=0.0, "Changed"=FALSE}, {"Status"="RW", "Name"="amplitude (V)", "Value"=0.0, "Changed"=FALSE}, {"Status"="RW", "Name"="phase dif (deg)", "Value"=0.0, "Changed"=FALSE}, {"Status"="RW", "Name"="sweep time (s)", "Value"=0.0, "Changed"=FALSE}, {"Status"="HVpuls1", "Name"="polarity (0=n)", "Value"=0.0, "Changed"=FALSE}, {"Status"="HVpuls1", "Name"="enable (0,1)", "Value"=0.0, "Changed"=FALSE}, {"Status"="HVpuls1", "Name"="amplitude (V)", "Value"=0.0, "Changed"=FALSE}, {"Status"="HVptime", "Name"="Mush on (0,1)", "Value"=0.0, "Changed"=FALSE}, {"Status"="HVptime", "Name"="Posi on (0,1)", "Value"=0.0, "Changed"=FALSE}, {"Status"="HVptime", "Name"="Cusp on (0,1)", "Value"=0.0, "Changed"=FALSE}, {"Status"="HVptime", "Name"="Posi width (s)", "Value"=0.0, "Changed"=FALSE}, {"Status"="HVptime", "Name"="Cusp delay (s)", "Value"=0.0, "Changed"=FALSE}, {"Status"="HVptime", "Name"="Cusp width (s)", "Value"=0.0, "Changed"=FALSE}, {"Status"="Dcoils", "Name"="Higaki A  (A)", "Value"=0.0, "Changed"=FALSE}, {"Status"="Dcoils", "Name"="Higaki B,C (A)", "Value"=0.0, "Changed"=FALSE}, {"Status"="Horn", "Name"="Klaxon (0,1)", "Value"=0.0, "Changed"=FALSE}, {"Status"="AMT", "Name"="posAMT (0,1)", "Value"=0.0, "Changed"=FALSE}, {"Status"="Scoop", "Name"="Acquisitions", "Value"=0.0, "Changed"=FALSE}, {"Status"="MCP", "Name"="front bias (V)", "Value"=0.0, "Changed"=FALSE}, {"Status"="MCP", "Name"="back bias (V)", "Value"=0.0, "Changed"=FALSE}, {"Status"="MCP", "Name"="phos bias (V)", "Value"=0.0, "Changed"=FALSE}, {"Status"="FI", "Name"="US bias (V)", "Value"=0.0, "Changed"=FALSE}, {"Status"="FI", "Name"="DS bias (V)", "Value"=0.0, "Changed"=FALSE}], "Comment"="downstream dump\nno ekick", "Reps"=10}, {"Toggle"=FALSE, "Open parameter editor"=FALSE, "Open MacroEditor"=FALSE, "Macro path"=path "C:/CuspControl/Cusp/1_Macros/Antiprotons/Reservoir/v102/scoopDS__014.mac", "Duration (s)"=0.094, "Parameters"=[{"Status"="ADC", "Name"="mode (0,1,2)", "Value"=0.0, "Changed"=FALSE}, {"Status"="Camera", "Name"="state (0,1)", "Value"=0.0, "Changed"=FALSE}, {"Status"="Slave", "Name"="state (0,1)", "Value"=0.0, "Changed"=FALSE}, {"Status"="Wait", "Name"="inbit (0...7)", "Value"=0.0, "Changed"=FALSE}, {"Status"="e-", "Name"="burn time (s)", "Value"=0.0, "Changed"=FALSE}, {"Status"="e-", "Name"="filament (A)", "Value"=0.0, "Changed"=FALSE}, {"Status"="e-", "Name"="enable (0,1)", "Value"=0.0, "Changed"=FALSE}, {"Status"="RW", "Name"="mode (0-13)", "Value"=0.0, "Changed"=FALSE}, {"Status"="RW", "Name"="f_start (Hz)", "Value"=0.0, "Changed"=FALSE}, {"Status"="RW", "Name"="f_stop (Hz)", "Value"=0.0, "Changed"=FALSE}, {"Status"="RW", "Name"="amplitude (V)", "Value"=0.0, "Changed"=FALSE}, {"Status"="RW", "Name"="phase dif (deg)", "Value"=0.0, "Changed"=FALSE}, {"Status"="RW", "Name"="sweep time (s)", "Value"=0.0, "Changed"=FALSE}, {"Status"="HVpuls1", "Name"="polarity (0=n)", "Value"=0.0, "Changed"=FALSE}, {"Status"="HVpuls1", "Name"="enable (0,1)", "Value"=0.0, "Changed"=FALSE}, {"Status"="HVpuls1", "Name"="amplitude (V)", "Value"=0.0, "Changed"=FALSE}, {"Status"="HVptime", "Name"="Mush on (0,1)", "Value"=0.0, "Changed"=FALSE}, {"Status"="HVptime", "Name"="Posi on (0,1)", "Value"=0.0, "Changed"=FALSE}, {"Status"="HVptime", "Name"="Cusp on (0,1)", "Value"=0.0, "Changed"=FALSE}, {"Status"="HVptime", "Name"="Posi width (s)", "Value"=0.0, "Changed"=FALSE}, {"Status"="HVptime", "Name"="Cusp delay (s)", "Value"=0.0, "Changed"=FALSE}, {"Status"="HVptime", "Name"="Cusp width (s)", "Value"=0.0, "Changed"=FALSE}, {"Status"="Dcoils", "Name"="Higaki A  (A)", "Value"=0.0, "Changed"=FALSE}, {"Status"="Dcoils", "Name"="Higaki B,C (A)", "Value"=0.0, "Changed"=FALSE}, {"Status"="Horn", "Name"="Klaxon (0,1)", "Value"=0.0, "Changed"=FALSE}, {"Status"="AMT", "Name"="posAMT (0,1)", "Value"=0.0, "Changed"=FALSE}, {"Status"="Scoop", "Name"="Acquisitions", "Value"=0.0, "Changed"=FALSE}, {"Status"="MCP", "Name"="front bias (V)", "Value"=0.0, "Changed"=FALSE}, {"Status"="MCP", "Name"="back bias (V)", "Value"=0.0, "Changed"=FALSE}, {"Status"="MCP", "Name"="phos bias (V)", "Value"=0.0, "Changed"=FALSE}, {"Status"="FI", "Name"="US bias (V)", "Value"=0.0, "Changed"=FALSE}, {"Status"="FI", "Name"="DS bias (V)", "Value"=0.0, "Changed"=FALSE}], "Comment"="downstream dump\nno ekick", "Reps"=10}, {"Toggle"=FALSE, "Open parameter editor"=FALSE, "Open MacroEditor"=FALSE, "Macro path"=path "C:/CuspControl/Cusp/1_Macros/Antiprotons/Reservoir/v102/scoopDS__015.mac", "Duration (s)"=0.094, "Parameters"=[{"Status"="ADC", "Name"="mode (0,1,2)", "Value"=0.0, "Changed"=FALSE}, {"Status"="Camera", "Name"="state (0,1)", "Value"=0.0, "Changed"=FALSE}, {"Status"="Slave", "Name"="state (0,1)", "Value"=0.0, "Changed"=FALSE}, {"Status"="Wait", "Name"="inbit (0...7)", "Value"=0.0, "Changed"=FALSE}, {"Status"="e-", "Name"="burn time (s)", "Value"=0.0, "Changed"=FALSE}, {"Status"="e-", "Name"="filament (A)", "Value"=0.0, "Changed"=FALSE}, {"Status"="e-", "Name"="enable (0,1)", "Value"=0.0, "Changed"=FALSE}, {"Status"="RW", "Name"="mode (0-13)", "Value"=0.0, "Changed"=FALSE}, {"Status"="RW", "Name"="f_start (Hz)", "Value"=0.0, "Changed"=FALSE}, {"Status"="RW", "Name"="f_stop (Hz)", "Value"=0.0, "Changed"=FALSE}, {"Status"="RW", "Name"="amplitude (V)", "Value"=0.0, "Changed"=FALSE}, {"Status"="RW", "Name"="phase dif (deg)", "Value"=0.0, "Changed"=FALSE}, {"Status"="RW", "Name"="sweep time (s)", "Value"=0.0, "Changed"=FALSE}, {"Status"="HVpuls1", "Name"="polarity (0=n)", "Value"=0.0, "Changed"=FALSE}, {"Status"="HVpuls1", "Name"="enable (0,1)", "Value"=0.0, "Changed"=FALSE}, {"Status"="HVpuls1", "Name"="amplitude (V)", "Value"=0.0, "Changed"=FALSE}, {"Status"="HVptime", "Name"="Mush on (0,1)", "Value"=0.0, "Changed"=FALSE}, {"Status"="HVptime", "Name"="Posi on (0,1)", "Value"=0.0, "Changed"=FALSE}, {"Status"="HVptime", "Name"="Cusp on (0,1)", "Value"=0.0, "Changed"=FALSE}, {"Status"="HVptime", "Name"="Posi width (s)", "Value"=0.0, "Changed"=FALSE}, {"Status"="HVptime", "Name"="Cusp delay (s)", "Value"=0.0, "Changed"=FALSE}, {"Status"="HVptime", "Name"="Cusp width (s)", "Value"=0.0, "Changed"=FALSE}, {"Status"="Dcoils", "Name"="Higaki A  (A)", "Value"=0.0, "Changed"=FALSE}, {"Status"="Dcoils", "Name"="Higaki B,C (A)", "Value"=0.0, "Changed"=FALSE}, {"Status"="Horn", "Name"="Klaxon (0,1)", "Value"=0.0, "Changed"=FALSE}, {"Status"="AMT", "Name"="posAMT (0,1)", "Value"=0.0, "Changed"=FALSE}, {"Status"="Scoop", "Name"="Acquisitions", "Value"=0.0, "Changed"=FALSE}, {"Status"="MCP", "Name"="front bias (V)", "Value"=0.0, "Changed"=FALSE}, {"Status"="MCP", "Name"="back bias (V)", "Value"=0.0, "Changed"=FALSE}, {"Status"="MCP", "Name"="phos bias (V)", "Value"=0.0, "Changed"=FALSE}, {"Status"="FI", "Name"="US bias (V)", "Value"=0.0, "Changed"=FALSE}, {"Status"="FI", "Name"="DS bias (V)", "Value"=0.0, "Changed"=FALSE}], "Comment"="downstream dump\nno ekick", "Reps"=10}, {"Toggle"=FALSE, "Open parameter editor"=FALSE, "Open MacroEditor"=FALSE, "Macro path"=path "C:/CuspControl/Cusp/1_Macros/Antiprotons/Reservoir/v102/scoopDS__016.mac", "Duration (s)"=0.094, "Parameters"=[{"Status"="ADC", "Name"="mode (0,1,2)", "Value"=0.0, "Changed"=FALSE}, {"Status"="Camera", "Name"="state (0,1)", "Value"=0.0, "Changed"=FALSE}, {"Status"="Slave", "Name"="state (0,1)", "Value"=0.0, "Changed"=FALSE}, {"Status"="Wait", "Name"="inbit (0...7)", "Value"=0.0, "Changed"=FALSE}, {"Status"="e-", "Name"="burn time (s)", "Value"=0.0, "Changed"=FALSE}, {"Status"="e-", "Name"="filament (A)", "Value"=0.0, "Changed"=FALSE}, {"Status"="e-", "Name"="enable (0,1)", "Value"=0.0, "Changed"=FALSE}, {"Status"="RW", "Name"="mode (0-13)", "Value"=0.0, "Changed"=FALSE}, {"Status"="RW", "Name"="f_start (Hz)", "Value"=0.0, "Changed"=FALSE}, {"Status"="RW", "Name"="f_stop (Hz)", "Value"=0.0, "Changed"=FALSE}, {"Status"="RW", "Name"="amplitude (V)", "Value"=0.0, "Changed"=FALSE}, {"Status"="RW", "Name"="phase dif (deg)", "Value"=0.0, "Changed"=FALSE}, {"Status"="RW", "Name"="sweep time (s)", "Value"=0.0, "Changed"=FALSE}, {"Status"="HVpuls1", "Name"="polarity (0=n)", "Value"=0.0, "Changed"=FALSE}, {"Status"="HVpuls1", "Name"="enable (0,1)", "Value"=0.0, "Changed"=FALSE}, {"Status"="HVpuls1", "Name"="amplitude (V)", "Value"=0.0, "Changed"=FALSE}, {"Status"="HVptime", "Name"="Mush on (0,1)", "Value"=0.0, "Changed"=FALSE}, {"Status"="HVptime", "Name"="Posi on (0,1)", "Value"=0.0, "Changed"=FALSE}, {"Status"="HVptime", "Name"="Cusp on (0,1)", "Value"=0.0, "Changed"=FALSE}, {"Status"="HVptime", "Name"="Posi width (s)", "Value"=0.0, "Changed"=FALSE}, {"Status"="HVptime", "Name"="Cusp delay (s)", "Value"=0.0, "Changed"=FALSE}, {"Status"="HVptime", "Name"="Cusp width (s)", "Value"=0.0, "Changed"=FALSE}, {"Status"="Dcoils", "Name"="Higaki A  (A)", "Value"=0.0, "Changed"=FALSE}, {"Status"="Dcoils", "Name"="Higaki B,C (A)", "Value"=0.0, "Changed"=FALSE}, {"Status"="Horn", "Name"="Klaxon (0,1)", "Value"=0.0, "Changed"=FALSE}, {"Status"="AMT", "Name"="posAMT (0,1)", "Value"=0.0, "Changed"=FALSE}, {"Status"="Scoop", "Name"="Acquisitions", "Value"=0.0, "Changed"=FALSE}, {"Status"="MCP", "Name"="front bias (V)", "Value"=0.0, "Changed"=FALSE}, {"Status"="MCP", "Name"="back bias (V)", "Value"=0.0, "Changed"=FALSE}, {"Status"="MCP", "Name"="phos bias (V)", "Value"=0.0, "Changed"=FALSE}, {"Status"="FI", "Name"="US bias (V)", "Value"=0.0, "Changed"=FALSE}, {"Status"="FI", "Name"="DS bias (V)", "Value"=0.0, "Changed"=FALSE}], "Comment"="downstream dump\nno ekick", "Reps"=10}, {"Toggle"=FALSE, "Open parameter editor"=FALSE, "Open MacroEditor"=FALSE, "Macro path"=path "C:/CuspControl/Cusp/1_Macros/Antiprotons/Reservoir/v102/scoopDS__017.mac", "Duration (s)"=0.094, "Parameters"=[{"Status"="ADC", "Name"="mode (0,1,2)", "Value"=0.0, "Changed"=FALSE}, {"Status"="Camera", "Name"="state (0,1)", "Value"=0.0, "Changed"=FALSE}, {"Status"="Slave", "Name"="state (0,1)", "Value"=0.0, "Changed"=FALSE}, {"Status"="Wait", "Name"="inbit (0...7)", "Value"=0.0, "Changed"=FALSE}, {"Status"="e-", "Name"="burn time (s)", "Value"=0.0, "Changed"=FALSE}, {"Status"="e-", "Name"="filament (A)", "Value"=0.0, "Changed"=FALSE}, {"Status"="e-", "Name"="enable (0,1)", "Value"=0.0, "Changed"=FALSE}, {"Status"="RW", "Name"="mode (0-13)", "Value"=0.0, "Changed"=FALSE}, {"Status"="RW", "Name"="f_start (Hz)", "Value"=0.0, "Changed"=FALSE}, {"Status"="RW", "Name"="f_stop (Hz)", "Value"=0.0, "Changed"=FALSE}, {"Status"="RW", "Name"="amplitude (V)", "Value"=0.0, "Changed"=FALSE}, {"Status"="RW", "Name"="phase dif (deg)", "Value"=0.0, "Changed"=FALSE}, {"Status"="RW", "Name"="sweep time (s)", "Value"=0.0, "Changed"=FALSE}, {"Status"="HVpuls1", "Name"="polarity (0=n)", "Value"=0.0, "Changed"=FALSE}, {"Status"="HVpuls1", "Name"="enable (0,1)", "Value"=0.0, "Changed"=FALSE}, {"Status"="HVpuls1", "Name"="amplitude (V)", "Value"=0.0, "Changed"=FALSE}, {"Status"="HVptime", "Name"="Mush on (0,1)", "Value"=0.0, "Changed"=FALSE}, {"Status"="HVptime", "Name"="Posi on (0,1)", "Value"=0.0, "Changed"=FALSE}, {"Status"="HVptime", "Name"="Cusp on (0,1)", "Value"=0.0, "Changed"=FALSE}, {"Status"="HVptime", "Name"="Posi width (s)", "Value"=0.0, "Changed"=FALSE}, {"Status"="HVptime", "Name"="Cusp delay (s)", "Value"=0.0, "Changed"=FALSE}, {"Status"="HVptime", "Name"="Cusp width (s)", "Value"=0.0, "Changed"=FALSE}, {"Status"="Dcoils", "Name"="Higaki A  (A)", "Value"=0.0, "Changed"=FALSE}, {"Status"="Dcoils", "Name"="Higaki B,C (A)", "Value"=0.0, "Changed"=FALSE}, {"Status"="Horn", "Name"="Klaxon (0,1)", "Value"=0.0, "Changed"=FALSE}, {"Status"="AMT", "Name"="posAMT (0,1)", "Value"=0.0, "Changed"=FALSE}, {"Status"="Scoop", "Name"="Acquisitions", "Value"=0.0, "Changed"=FALSE}, {"Status"="MCP", "Name"="front bias (V)", "Value"=0.0, "Changed"=FALSE}, {"Status"="MCP", "Name"="back bias (V)", "Value"=0.0, "Changed"=FALSE}, {"Status"="MCP", "Name"="phos bias (V)", "Value"=0.0, "Changed"=FALSE}, {"Status"="FI", "Name"="US bias (V)", "Value"=0.0, "Changed"=FALSE}, {"Status"="FI", "Name"="DS bias (V)", "Value"=0.0, "Changed"=FALSE}], "Comment"="downstream dump\nno ekick", "Reps"=10}, {"Toggle"=FALSE, "Open parameter editor"=FALSE, "Open MacroEditor"=FALSE, "Macro path"=path "C:/CuspControl/Cusp/1_Macros/Antiprotons/Reservoir/v102/scoopDS__018.mac", "Duration (s)"=0.094, "Parameters"=[{"Status"="ADC", "Name"="mode (0,1,2)", "Value"=0.0, "Changed"=FALSE}, {"Status"="Camera", "Name"="state (0,1)", "Value"=0.0, "Changed"=FALSE}, {"Status"="Slave", "Name"="state (0,1)", "Value"=0.0, "Changed"=FALSE}, {"Status"="Wait", "Name"="inbit (0...7)", "Value"=0.0, "Changed"=FALSE}, {"Status"="e-", "Name"="burn time (s)", "Value"=0.0, "Changed"=FALSE}, {"Status"="e-", "Name"="filament (A)", "Value"=0.0, "Changed"=FALSE}, {"Status"="e-", "Name"="enable (0,1)", "Value"=0.0, "Changed"=FALSE}, {"Status"="RW", "Name"="mode (0-13)", "Value"=0.0, "Changed"=FALSE}, {"Status"="RW", "Name"="f_start (Hz)", "Value"=0.0, "Changed"=FALSE}, {"Status"="RW", "Name"="f_stop (Hz)", "Value"=0.0, "Changed"=FALSE}, {"Status"="RW", "Name"="amplitude (V)", "Value"=0.0, "Changed"=FALSE}, {"Status"="RW", "Name"="phase dif (deg)", "Value"=0.0, "Changed"=FALSE}, {"Status"="RW", "Name"="sweep time (s)", "Value"=0.0, "Changed"=FALSE}, {"Status"="HVpuls1", "Name"="polarity (0=n)", "Value"=0.0, "Changed"=FALSE}, {"Status"="HVpuls1", "Name"="enable (0,1)", "Value"=0.0, "Changed"=FALSE}, {"Status"="HVpuls1", "Name"="amplitude (V)", "Value"=0.0, "Changed"=FALSE}, {"Status"="HVptime", "Name"="Mush on (0,1)", "Value"=0.0, "Changed"=FALSE}, {"Status"="HVptime", "Name"="Posi on (0,1)", "Value"=0.0, "Changed"=FALSE}, {"Status"="HVptime", "Name"="Cusp on (0,1)", "Value"=0.0, "Changed"=FALSE}, {"Status"="HVptime", "Name"="Posi width (s)", "Value"=0.0, "Changed"=FALSE}, {"Status"="HVptime", "Name"="Cusp delay (s)", "Value"=0.0, "Changed"=FALSE}, {"Status"="HVptime", "Name"="Cusp width (s)", "Value"=0.0, "Changed"=FALSE}, {"Status"="Dcoils", "Name"="Higaki A  (A)", "Value"=0.0, "Changed"=FALSE}, {"Status"="Dcoils", "Name"="Higaki B,C (A)", "Value"=0.0, "Changed"=FALSE}, {"Status"="Horn", "Name"="Klaxon (0,1)", "Value"=0.0, "Changed"=FALSE}, {"Status"="AMT", "Name"="posAMT (0,1)", "Value"=0.0, "Changed"=FALSE}, {"Status"="Scoop", "Name"="Acquisitions", "Value"=0.0, "Changed"=FALSE}, {"Status"="MCP", "Name"="front bias (V)", "Value"=0.0, "Changed"=FALSE}, {"Status"="MCP", "Name"="back bias (V)", "Value"=0.0, "Changed"=FALSE}, {"Status"="MCP", "Name"="phos bias (V)", "Value"=0.0, "Changed"=FALSE}, {"Status"="FI", "Name"="US bias (V)", "Value"=0.0, "Changed"=FALSE}, {"Status"="FI", "Name"="DS bias (V)", "Value"=0.0, "Changed"=FALSE}], "Comment"="downstream dump\nno ekick", "Reps"=10}, {"Toggle"=FALSE, "Open parameter editor"=FALSE, "Open MacroEditor"=FALSE, "Macro path"=path "C:/CuspControl/Cusp/1_Macros/Antiprotons/Reservoir/v102/scoopDS__019.mac", "Duration (s)"=0.094, "Parameters"=[{"Status"="ADC", "Name"="mode (0,1,2)", "Value"=0.0, "Changed"=FALSE}, {"Status"="Camera", "Name"="state (0,1)", "Value"=0.0, "Changed"=FALSE}, {"Status"="Slave", "Name"="state (0,1)", "Value"=0.0, "Changed"=FALSE}, {"Status"="Wait", "Name"="inbit (0...7)", "Value"=0.0, "Changed"=FALSE}, {"Status"="e-", "Name"="burn time (s)", "Value"=0.0, "Changed"=FALSE}, {"Status"="e-", "Name"="filament (A)", "Value"=0.0, "Changed"=FALSE}, {"Status"="e-", "Name"="enable (0,1)", "Value"=0.0, "Changed"=FALSE}, {"Status"="RW", "Name"="mode (0-13)", "Value"=0.0, "Changed"=FALSE}, {"Status"="RW", "Name"="f_start (Hz)", "Value"=0.0, "Changed"=FALSE}, {"Status"="RW", "Name"="f_stop (Hz)", "Value"=0.0, "Changed"=FALSE}, {"Status"="RW", "Name"="amplitude (V)", "Value"=0.0, "Changed"=FALSE}, {"Status"="RW", "Name"="phase dif (deg)", "Value"=0.0, "Changed"=FALSE}, {"Status"="RW", "Name"="sweep time (s)", "Value"=0.0, "Changed"=FALSE}, {"Status"="HVpuls1", "Name"="polarity (0=n)", "Value"=0.0, "Changed"=FALSE}, {"Status"="HVpuls1", "Name"="enable (0,1)", "Value"=0.0, "Changed"=FALSE}, {"Status"="HVpuls1", "Name"="amplitude (V)", "Value"=0.0, "Changed"=FALSE}, {"Status"="HVptime", "Name"="Mush on (0,1)", "Value"=0.0, "Changed"=FALSE}, {"Status"="HVptime", "Name"="Posi on (0,1)", "Value"=0.0, "Changed"=FALSE}, {"Status"="HVptime", "Name"="Cusp on (0,1)", "Value"=0.0, "Changed"=FALSE}, {"Status"="HVptime", "Name"="Posi width (s)", "Value"=0.0, "Changed"=FALSE}, {"Status"="HVptime", "Name"="Cusp delay (s)", "Value"=0.0, "Changed"=FALSE}, {"Status"="HVptime", "Name"="Cusp width (s)", "Value"=0.0, "Changed"=FALSE}, {"Status"="Dcoils", "Name"="Higaki A  (A)", "Value"=0.0, "Changed"=FALSE}, {"Status"="Dcoils", "Name"="Higaki B,C (A)", "Value"=0.0, "Changed"=FALSE}, {"Status"="Horn", "Name"="Klaxon (0,1)", "Value"=0.0, "Changed"=FALSE}, {"Status"="AMT", "Name"="posAMT (0,1)", "Value"=0.0, "Changed"=FALSE}, {"Status"="Scoop", "Name"="Acquisitions", "Value"=0.0, "Changed"=FALSE}, {"Status"="MCP", "Name"="front bias (V)", "Value"=0.0, "Changed"=FALSE}, {"Status"="MCP", "Name"="back bias (V)", "Value"=0.0, "Changed"=FALSE}, {"Status"="MCP", "Name"="phos bias (V)", "Value"=0.0, "Changed"=FALSE}, {"Status"="FI", "Name"="US bias (V)", "Value"=0.0, "Changed"=FALSE}, {"Status"="FI", "Name"="DS bias (V)", "Value"=0.0, "Changed"=FALSE}], "Comment"="downstream dump\nno ekick", "Reps"=10}, {"Toggle"=FALSE, "Open parameter editor"=FALSE, "Open MacroEditor"=FALSE, "Macro path"=path "C:/CuspControl/Cusp/1_Macros/Antiprotons/Reservoir/v102/scoopDS__020.mac", "Duration (s)"=0.094, "Parameters"=[{"Status"="ADC", "Name"="mode (0,1,2)", "Value"=0.0, "Changed"=FALSE}, {"Status"="Camera", "Name"="state (0,1)", "Value"=0.0, "Changed"=FALSE}, {"Status"="Slave", "Name"="state (0,1)", "Value"=0.0, "Changed"=FALSE}, {"Status"="Wait", "Name"="inbit (0...7)", "Value"=0.0, "Changed"=FALSE}, {"Status"="e-", "Name"="burn time (s)", "Value"=0.0, "Changed"=FALSE}, {"Status"="e-", "Name"="filament (A)", "Value"=0.0, "Changed"=FALSE}, {"Status"="e-", "Name"="enable (0,1)", "Value"=0.0, "Changed"=FALSE}, {"Status"="RW", "Name"="mode (0-13)", "Value"=0.0, "Changed"=FALSE}, {"Status"="RW", "Name"="f_start (Hz)", "Value"=0.0, "Changed"=FALSE}, {"Status"="RW", "Name"="f_stop (Hz)", "Value"=0.0, "Changed"=FALSE}, {"Status"="RW", "Name"="amplitude (V)", "Value"=0.0, "Changed"=FALSE}, {"Status"="RW", "Name"="phase dif (deg)", "Value"=0.0, "Changed"=FALSE}, {"Status"="RW", "Name"="sweep time (s)", "Value"=0.0, "Changed"=FALSE}, {"Status"="HVpuls1", "Name"="polarity (0=n)", "Value"=0.0, "Changed"=FALSE}, {"Status"="HVpuls1", "Name"="enable (0,1)", "Value"=0.0, "Changed"=FALSE}, {"Status"="HVpuls1", "Name"="amplitude (V)", "Value"=0.0, "Changed"=FALSE}, {"Status"="HVptime", "Name"="Mush on (0,1)", "Value"=0.0, "Changed"=FALSE}, {"Status"="HVptime", "Name"="Posi on (0,1)", "Value"=0.0, "Changed"=FALSE}, {"Status"="HVptime", "Name"="Cusp on (0,1)", "Value"=0.0, "Changed"=FALSE}, {"Status"="HVptime", "Name"="Posi width (s)", "Value"=0.0, "Changed"=FALSE}, {"Status"="HVptime", "Name"="Cusp delay (s)", "Value"=0.0, "Changed"=FALSE}, {"Status"="HVptime", "Name"="Cusp width (s)", "Value"=0.0, "Changed"=FALSE}, {"Status"="Dcoils", "Name"="Higaki A  (A)", "Value"=0.0, "Changed"=FALSE}, {"Status"="Dcoils", "Name"="Higaki B,C (A)", "Value"=0.0, "Changed"=FALSE}, {"Status"="Horn", "Name"="Klaxon (0,1)", "Value"=0.0, "Changed"=FALSE}, {"Status"="AMT", "Name"="posAMT (0,1)", "Value"=0.0, "Changed"=FALSE}, {"Status"="Scoop", "Name"="Acquisitions", "Value"=0.0, "Changed"=FALSE}, {"Status"="MCP", "Name"="front bias (V)", "Value"=0.0, "Changed"=FALSE}, {"Status"="MCP", "Name"="back bias (V)", "Value"=0.0, "Changed"=FALSE}, {"Status"="MCP", "Name"="phos bias (V)", "Value"=0.0, "Changed"=FALSE}, {"Status"="FI", "Name"="US bias (V)", "Value"=0.0, "Changed"=FALSE}, {"Status"="FI", "Name"="DS bias (V)", "Value"=0.0, "Changed"=FALSE}], "Comment"="downstream dump\nno ekick", "Reps"=10}] {"Reps" min=1 step=1; "Parameters"."Value" format="%_6p"; "Duration (s)" min=0.001 step=0.001 format="%_6p"}
  in  "stop":bool
  in  "Save":bool=TRUE
  in  "Save/Open Path":path=path "C:/CuspControl/Cusp/1_Cues/Test/2026-04-23/Manymacros.q"
  in  "Open":bool
  in  "New":bool
  out "# Actions":i32=22
  in  "Cue Description":string
  out "Total Time (s)":dbl=19.750000000000004 format="%.3f"
  in  "System":u16(ring) items=["Cusp", "Positron", "Musashi"]
  out "InfoArray":cluster{"Action":i32, "Time":dbl}[](array[cluster])=[{"Action"=0, "Time"=0.0}, {"Action"=1, "Time"=0.01}, {"Action"=2, "Time"=0.95}, {"Action"=3, "Time"=1.89}, {"Action"=4, "Time"=2.83}, {"Action"=5, "Time"=3.77}, {"Action"=6, "Time"=4.71}, {"Action"=7, "Time"=5.65}, {"Action"=8, "Time"=6.59}, {"Action"=9, "Time"=7.529999999999999}, {"Action"=10, "Time"=8.469999999999999}, {"Action"=11, "Time"=9.409999999999998}, {"Action"=12, "Time"=10.349999999999998}, {"Action"=13, "Time"=11.289999999999997}, {"Action"=14, "Time"=12.229999999999997}, {"Action"=15, "Time"=13.169999999999996}, {"Action"=16, "Time"=14.109999999999996}, {"Action"=17, "Time"=15.049999999999995}, {"Action"=18, "Time"=15.989999999999995}, {"Action"=19, "Time"=16.929999999999996}, {"Action"=20, "Time"=17.869999999999997}, {"Action"=21, "Time"=18.81}] {"Time" format="%.3f"}
  in  "Params paths":path[](array[path])=[path "C:/CuspControl/Cusp/Configuration/Parameters.txt", path "C:/CuspControl/Positron/Configuration/Parameters.txt", path "C:/CuspControl/Musashi/Configuration/Parameters.txt"]
  in  "Default Parameters":T3=[{"Status"="ADC", "Name"="mode (0,1,2)", "Value"=0.0, "Changed"=FALSE}, {"Status"="Camera", "Name"="state (0,1)", "Value"=0.0, "Changed"=FALSE}, {"Status"="Slave", "Name"="state (0,1)", "Value"=0.0, "Changed"=FALSE}, {"Status"="Wait", "Name"="inbit (0...7)", "Value"=0.0, "Changed"=FALSE}, {"Status"="e-", "Name"="burn time (s)", "Value"=0.0, "Changed"=FALSE}, {"Status"="e-", "Name"="filament (A)", "Value"=0.0, "Changed"=FALSE}, {"Status"="e-", "Name"="enable (0,1)", "Value"=0.0, "Changed"=FALSE}, {"Status"="RW", "Name"="mode (0-13)", "Value"=0.0, "Changed"=FALSE}, {"Status"="RW", "Name"="f_start (Hz)", "Value"=0.0, "Changed"=FALSE}, {"Status"="RW", "Name"="f_stop (Hz)", "Value"=0.0, "Changed"=FALSE}, {"Status"="RW", "Name"="amplitude (V)", "Value"=0.0, "Changed"=FALSE}, {"Status"="RW", "Name"="phase dif (deg)", "Value"=0.0, "Changed"=FALSE}, {"Status"="RW", "Name"="sweep time (s)", "Value"=0.0, "Changed"=FALSE}, {"Status"="HVpuls1", "Name"="polarity (0=n)", "Value"=0.0, "Changed"=FALSE}, {"Status"="HVpuls1", "Name"="enable (0,1)", "Value"=0.0, "Changed"=FALSE}, {"Status"="HVpuls1", "Name"="amplitude (V)", "Value"=0.0, "Changed"=FALSE}, {"Status"="HVptime", "Name"="Mush on (0,1)", "Value"=0.0, "Changed"=FALSE}, {"Status"="HVptime", "Name"="Posi on (0,1)", "Value"=0.0, "Changed"=FALSE}, {"Status"="HVptime", "Name"="Cusp on (0,1)", "Value"=0.0, "Changed"=FALSE}, {"Status"="HVptime", "Name"="Posi width (s)", "Value"=0.0, "Changed"=FALSE}, {"Status"="HVptime", "Name"="Cusp delay (s)", "Value"=0.0, "Changed"=FALSE}, {"Status"="HVptime", "Name"="Cusp width (s)", "Value"=0.0, "Changed"=FALSE}, {"Status"="Dcoils", "Name"="Higaki A  (A)", "Value"=0.0, "Changed"=FALSE}, {"Status"="Dcoils", "Name"="Higaki B,C (A)", "Value"=0.0, "Changed"=FALSE}, {"Status"="Horn", "Name"="Klaxon (0,1)", "Value"=0.0, "Changed"=FALSE}, {"Status"="AMT", "Name"="posAMT (0,1)", "Value"=0.0, "Changed"=FALSE}, {"Status"="Scoop", "Name"="Acquisitions", "Value"=0.0, "Changed"=FALSE}, {"Status"="MCP", "Name"="front bias (V)", "Value"=0.0, "Changed"=FALSE}, {"Status"="MCP", "Name"="back bias (V)", "Value"=0.0, "Changed"=FALSE}, {"Status"="MCP", "Name"="phos bias (V)", "Value"=0.0, "Changed"=FALSE}, {"Status"="FI", "Name"="US bias (V)", "Value"=0.0, "Changed"=FALSE}, {"Status"="FI", "Name"="DS bias (V)", "Value"=0.0, "Changed"=FALSE}] {"Value" format="%_6p"}
  out "Default Action":T2={"Toggle"=TRUE, "Open parameter editor"=FALSE, "Open MacroEditor"=FALSE, "Macro path"=path "", "Duration (s)"=0.001, "Parameters"=[{"Status"="ADC", "Name"="mode (0,1,2)", "Value"=0.0, "Changed"=FALSE}, {"Status"="Camera", "Name"="state (0,1)", "Value"=0.0, "Changed"=FALSE}, {"Status"="Slave", "Name"="state (0,1)", "Value"=0.0, "Changed"=FALSE}, {"Status"="Wait", "Name"="inbit (0...7)", "Value"=0.0, "Changed"=FALSE}, {"Status"="e-", "Name"="burn time (s)", "Value"=0.0, "Changed"=FALSE}, {"Status"="e-", "Name"="filament (A)", "Value"=0.0, "Changed"=FALSE}, {"Status"="e-", "Name"="enable (0,1)", "Value"=0.0, "Changed"=FALSE}, {"Status"="RW", "Name"="mode (0-13)", "Value"=0.0, "Changed"=FALSE}, {"Status"="RW", "Name"="f_start (Hz)", "Value"=0.0, "Changed"=FALSE}, {"Status"="RW", "Name"="f_stop (Hz)", "Value"=0.0, "Changed"=FALSE}, {"Status"="RW", "Name"="amplitude (V)", "Value"=0.0, "Changed"=FALSE}, {"Status"="RW", "Name"="phase dif (deg)", "Value"=0.0, "Changed"=FALSE}, {"Status"="RW", "Name"="sweep time (s)", "Value"=0.0, "Changed"=FALSE}, {"Status"="HVpuls1", "Name"="polarity (0=n)", "Value"=0.0, "Changed"=FALSE}, {"Status"="HVpuls1", "Name"="enable (0,1)", "Value"=0.0, "Changed"=FALSE}, {"Status"="HVpuls1", "Name"="amplitude (V)", "Value"=0.0, "Changed"=FALSE}, {"Status"="HVptime", "Name"="Mush on (0,1)", "Value"=0.0, "Changed"=FALSE}, {"Status"="HVptime", "Name"="Posi on (0,1)", "Value"=0.0, "Changed"=FALSE}, {"Status"="HVptime", "Name"="Cusp on (0,1)", "Value"=0.0, "Changed"=FALSE}, {"Status"="HVptime", "Name"="Posi width (s)", "Value"=0.0, "Changed"=FALSE}, {"Status"="HVptime", "Name"="Cusp delay (s)", "Value"=0.0, "Changed"=FALSE}, {"Status"="HVptime", "Name"="Cusp width (s)", "Value"=0.0, "Changed"=FALSE}, {"Status"="Dcoils", "Name"="Higaki A  (A)", "Value"=0.0, "Changed"=FALSE}, {"Status"="Dcoils", "Name"="Higaki B,C (A)", "Value"=0.0, "Changed"=FALSE}, {"Status"="Horn", "Name"="Klaxon (0,1)", "Value"=0.0, "Changed"=FALSE}, {"Status"="AMT", "Name"="posAMT (0,1)", "Value"=0.0, "Changed"=FALSE}, {"Status"="Scoop", "Name"="Acquisitions", "Value"=0.0, "Changed"=FALSE}, {"Status"="MCP", "Name"="front bias (V)", "Value"=0.0, "Changed"=FALSE}, {"Status"="MCP", "Name"="back bias (V)", "Value"=0.0, "Changed"=FALSE}, {"Status"="MCP", "Name"="phos bias (V)", "Value"=0.0, "Changed"=FALSE}, {"Status"="FI", "Name"="US bias (V)", "Value"=0.0, "Changed"=FALSE}, {"Status"="FI", "Name"="DS bias (V)", "Value"=0.0, "Changed"=FALSE}], "Comment"="", "Reps"=10} {"Reps" min=1 step=1; "Parameters"."Value" format="%_6p"; "Duration (s)" min=0.001 step=0.001 format="%_6p"}
  out "Params list":string[][](array[string])=[["ADC", "mode (0,1,2)", "txt", "C:\\CuspControl\\GPIB and Network\\Cusp\\ADCState.txt", "", "", "", ""], ["Camera", "state (0,1)", "txt", "C:\\CuspControl\\GPIB and Network\\Cusp\\CameraState.txt", "", "", "", ""], ["Slave", "state (0,1)", "txt", "C:\\CuspControl\\GPIB and Network\\Cusp\\SlaveState.txt", "", "", "", ""], ["Wait", "inbit (0...7)", "dac", "0.1", "inbit", "-1", "0", "7"], ["e-", "burn time (s)", "txt", "C:\\CuspControl\\GPIB and Network\\Cusp\\esourceRampVoltandState.txt", "", "", "", ""], ["e-", "filament (A)", "txt", "C:\\CuspControl\\GPIB and Network\\Cusp\\esourceRampVoltandState.txt", "", "", "", ""], ["e-", "enable (0,1)", "txt", "C:\\CuspControl\\GPIB and Network\\Cusp\\esourceRampVoltandState.txt", "", "", "", ""], ["RW", "mode (0-13)", "txt", "C:\\CuspControl\\GPIB and Network\\Cusp\\RWparams.txt", "", "", "", ""], ["RW", "f_start (Hz)", "txt", "C:\\CuspControl\\GPIB and Network\\Cusp\\RWparams.txt", "", "", "", ""], ["RW", "f_stop (Hz)", "txt", "C:\\CuspControl\\GPIB and Network\\Cusp\\RWparams.txt", "", "", "", ""], ["RW", "amplitude (V)", "txt", "C:\\CuspControl\\GPIB and Network\\Cusp\\RWparams.txt", "", "", "", ""], ["RW", "phase dif (deg)", "txt", "C:\\CuspControl\\GPIB and Network\\Cusp\\RWparams.txt", "", "", "", ""], ["RW", "sweep time (s)", "txt", "C:\\CuspControl\\GPIB and Network\\Cusp\\RWparams.txt", "", "", "", ""], ["HVpuls1", "polarity (0=n)", "dac", "0.1", "ao0", "0.2", "0", "1"], ["HVpuls1", "enable (0,1)", "dac", "0.1", "ao1", "0.1", "0", "1"], ["HVpuls1", "amplitude (V)", "dac", "0.1", "ao2", "15", "0", "110"], ["HVptime", "Mush on (0,1)", "txt", "C:\\CuspControl\\GPIB and Network\\Cusp\\HVpulseTiming.txt", "", "", "", ""], ["HVptime", "Posi on (0,1)", "txt", "C:\\CuspControl\\GPIB and Network\\Cusp\\HVpulseTiming.txt", "", "", "", ""], ["HVptime", "Cusp on (0,1)", "txt", "C:\\CuspControl\\GPIB and Network\\Cusp\\HVpulseTiming.txt", "", "", "", ""], ["HVptime", "Posi width (s)", "txt", "C:\\CuspControl\\GPIB and Network\\Cusp\\HVpulseTiming.txt", "", "", "", ""], ["HVptime", "Cusp delay (s)", "txt", "C:\\CuspControl\\GPIB and Network\\Cusp\\HVpulseTiming.txt", "", "", "", ""], ["HVptime", "Cusp width (s)", "txt", "C:\\CuspControl\\GPIB and Network\\Cusp\\HVpulseTiming.txt", "", "", "", ""], ["Dcoils", "Higaki A  (A)", "dac", "0.5", "ao8", "12", "0", "60"], ["Dcoils", "Higaki B,C (A)", "dac", "0.5", "ao9", "9", "0", "45"], ["Horn", "Klaxon (0,1)", "txt", "C:\\CuspControl\\GPIB and Network\\Cusp\\Klaxon.txt", "", "", "", ""], ["AMT", "posAMT (0,1)", "txt", "C:\\CuspControl\\GPIB and Network\\Cusp\\posAMT.txt", "", "", "", ""], ["Scoop", "Acquisitions", "txt", "C:\\CuspControl\\GPIB and Network\\Cusp\\ScoopAcqs.txt", "", "", "", ""], ["MCP", "front bias (V)", "dac", "4.0", "ao5", "15", "-130", "130"], ["MCP", "back bias (V)", "dac", "4.0", "ao6", "200", "0", "1000"], ["MCP", "phos bias (V)", "dac", "4.0", "ao7", "500", "0", "3500"], ["FI", "US bias (V)", "dac", "1.0", "ao10", "200", "0", "800"], ["FI", "DS bias (V)", "dac", "1.0", "ao11", "200", "0", "800"]]
  in  "Param Buffer (200 ms)":dbl format="%#_3p"
  out "LastMods":timestamp[](array[timestamp])=[timestamp(0 s since 1904-01-01), timestamp(3845449783 s since 1904-01-01), timestamp(3845449783 s since 1904-01-01), timestamp(3845449783 s since 1904-01-01), timestamp(3845449783 s since 1904-01-01), timestamp(3845449783 s since 1904-01-01), timestamp(3845449783 s since 1904-01-01), timestamp(3845449783 s since 1904-01-01), timestamp(3845449783 s since 1904-01-01), timestamp(3845449783 s since 1904-01-01), timestamp(3845449783 s since 1904-01-01), timestamp(3845449783 s since 1904-01-01), timestamp(3845449783 s since 1904-01-01), timestamp(3845449783 s since 1904-01-01), timestamp(3845449783 s since 1904-01-01), timestamp(3845449783 s since 1904-01-01), timestamp(3845449783 s since 1904-01-01), timestamp(3845449783 s since 1904-01-01), timestamp(3845449783 s since 1904-01-01), timestamp(3845449783 s since 1904-01-01), timestamp(3845449783 s since 1904-01-01), timestamp(3845449783 s since 1904-01-01)]
  in  "US+DS":bool
  in  "Insert at Action":i32=1
  in  "Replace":bool
  in  "Add macros":bool
  in  "To end":bool
  in  "Last file":path=path "C:/CuspControl/Cusp/1_Macros/Antiprotons/Reservoir/v102/scoopDS__020.mac"
  in  "First file":path=path "C:/CuspControl/Cusp/1_Macros/Antiprotons/Reservoir/v102/scoopDS__000.mac"
  in  "US/DS":bool
  out "Last Value":i32=22
  out "Edit #":i32=-1
  # "browse"
  # "browse"
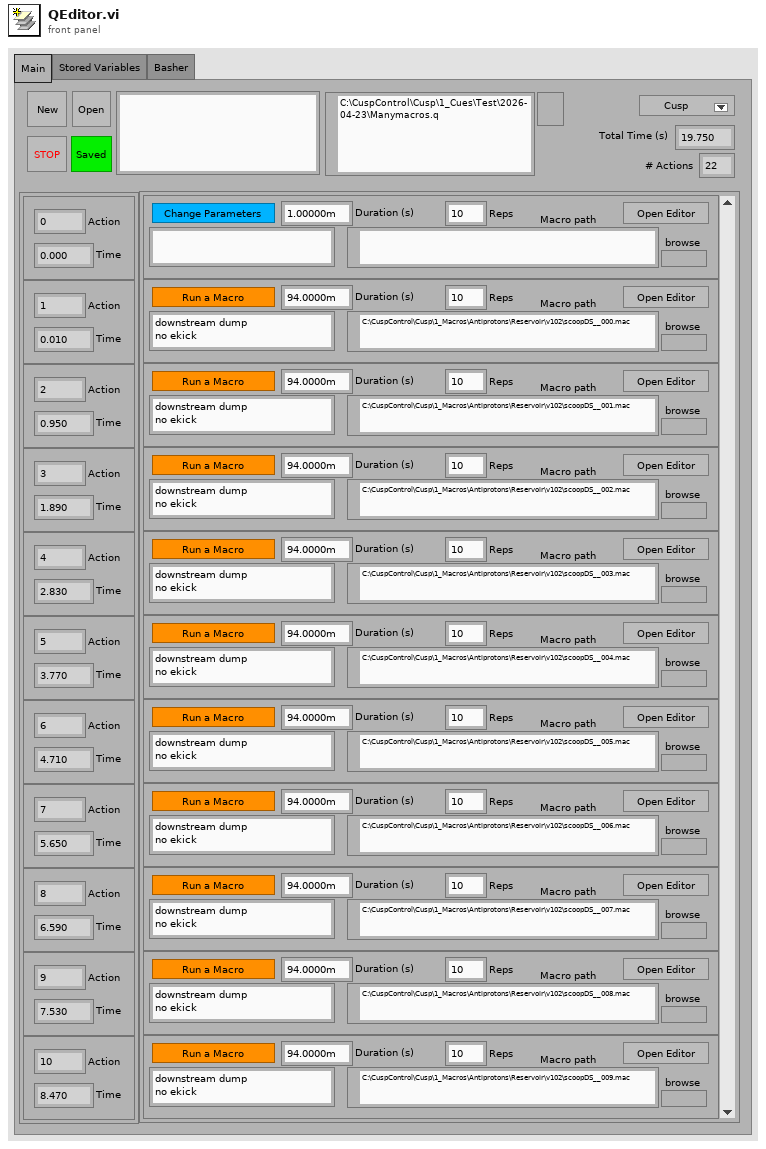
[diagram p1: front panel]
types:
  T1 = typedef "Actions_arr.ctl" = T2[]
  T2 = typedef "Action.ctl" = cluster{"Toggle":bool, "Open parameter editor":bool, "Open MacroEditor":bool, "Macro path":path, "Duration (s)":dbl, "Parameters":T3, "Comment":string, "Reps":i32}
  T3 = typedef "Parameters.ctl" = cluster{"Status":string, "Name":string, "Value":dbl, "Changed":bool}[]
  T4 = cluster{"Status":string, "Name":string, "Value":dbl, "Changed":bool}
  T5 = typedef "MacroSaveCluster.ctl" = cluster{"Instructions":T6, "Changes":bool[][], "Macro Description":string, "Total Time (s)":dbl, "Samples per sec":dbl}
  T6 = typedef "Instructions.ctl" = T7[]
  T7 = typedef "Instruction.ctl" = cluster{"Duration":dbl, "Comment":string, "Steps":i32, "Edit Potential":bool, "Output Bits":bool[], "Macro Path":path, "Potentials":dbl[], "Inherit?":bool}
  T8 = cluster{"Total Time (s)":dbl, "Cue Description":string}
  T9 = cluster{"Total\nTime (s)":dbl, "Cue Description":string}
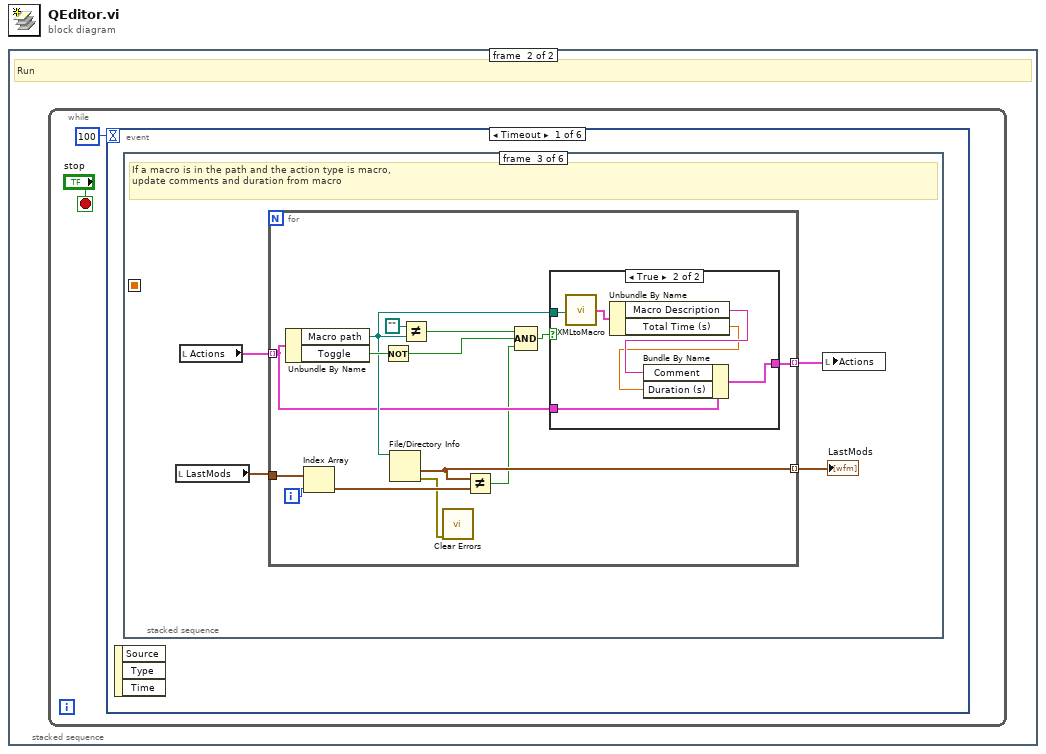
[diagram p0: block diagram]
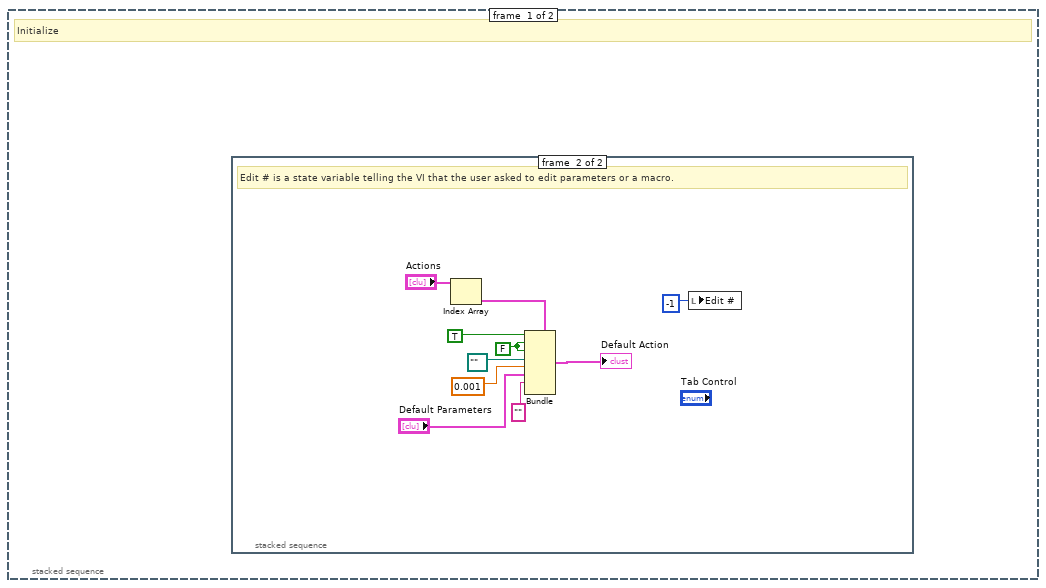
[diagram p2: hidden frame]
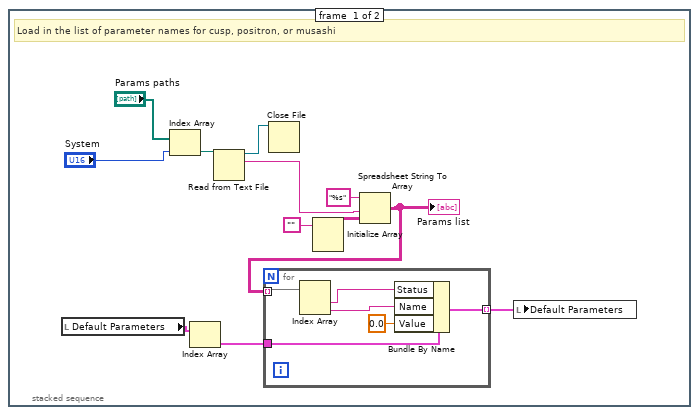
[diagram p3: hidden frame]
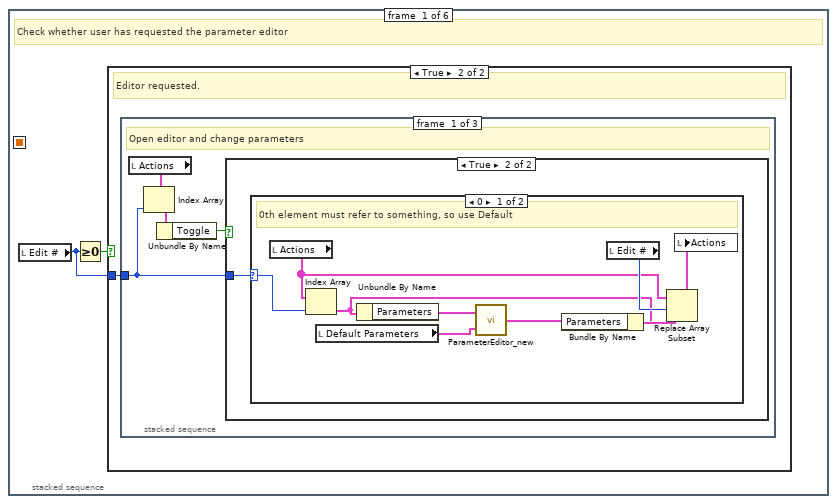
[diagram p4: hidden frame]
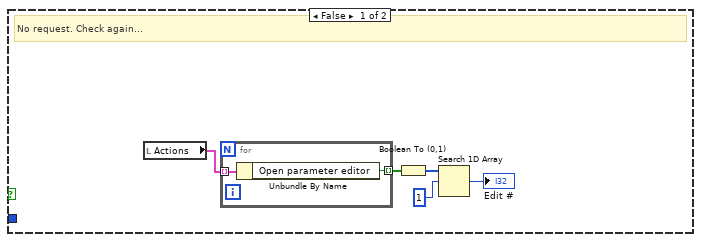
[diagram p5: hidden frame]
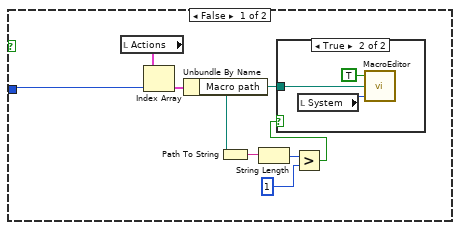
[diagram p6: hidden frame]
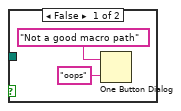
[diagram p7: hidden frame]
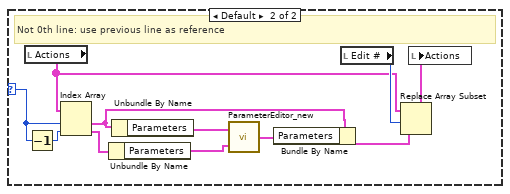
[diagram p8: hidden frame]
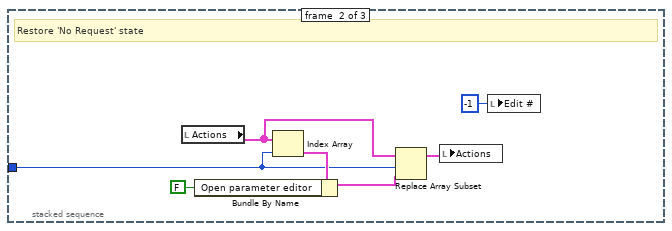
[diagram p9: hidden frame]
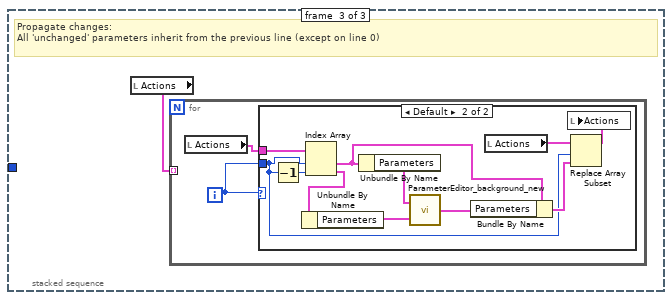
[diagram p10: hidden frame]
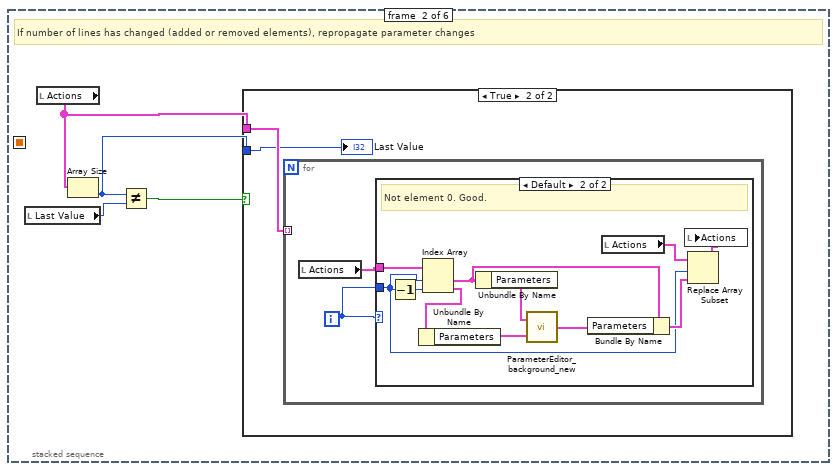
[diagram p12: hidden frame]
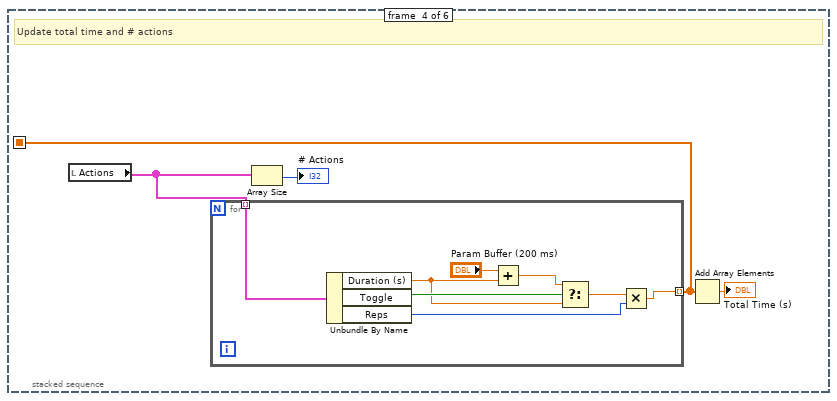
[diagram p16: hidden frame]
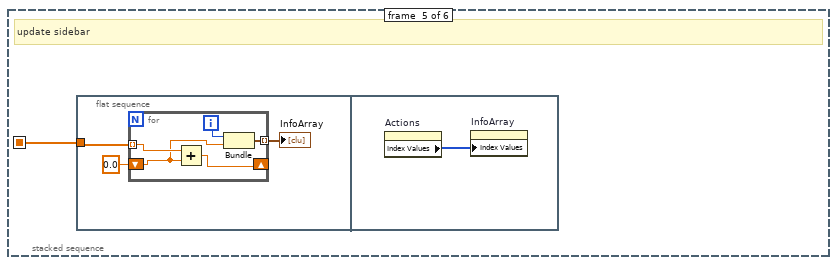
[diagram p17: hidden frame]
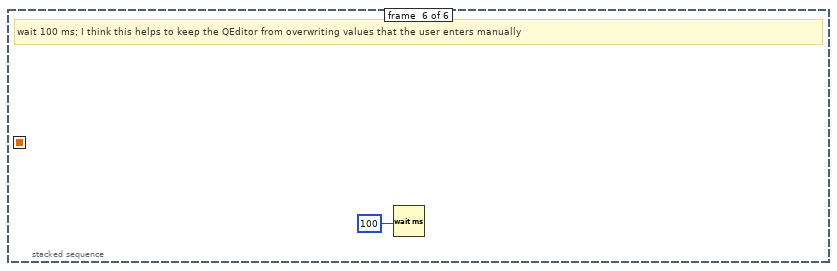
[diagram p18: hidden frame]
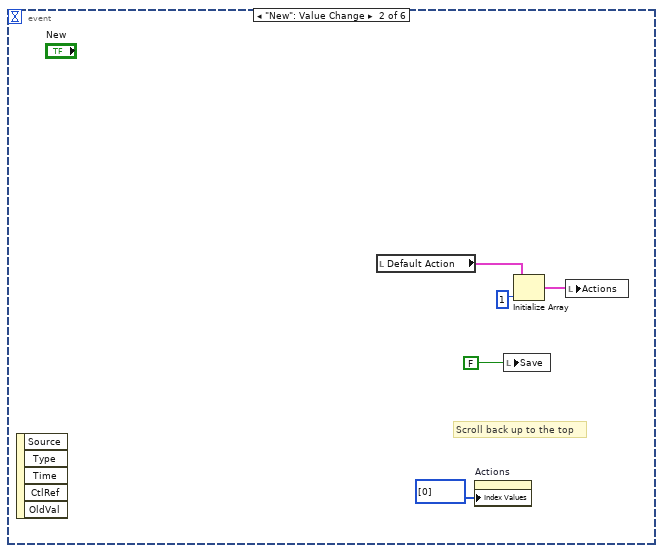
[diagram p19: hidden frame]
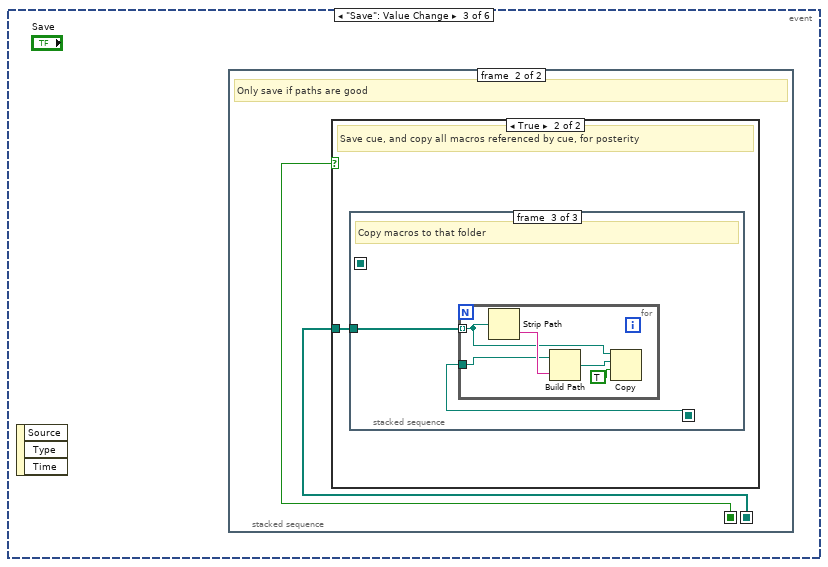
[diagram p20: hidden frame]
diagram:
  n1 = stacked-sequence {
    frame #0 {
      # "Initialize"
      n2 = stacked-sequence {
        frame #0 {
          # "Load in the list of parameter names for cusp, positron, or musashi"
          n3 = local read "Default Parameters"() -> (w5:T3)
          n4 = Index Array(array="Params paths", index="System") -> (element=w6:path)
          n5 = Index Array(array=w5) -> (element=w4:T4)  [unwired: 1 in]
          n6 = Read from Text File(file (use dialog)=w6) -> (refnum out=w7:refnum<file>, text=w9:string)  [unwired: 3 in, 2 out]
          n7 = Close File(refnum=w7) -> ()  [unwired: 1 in, 2 out]
          n8 = Initialize Array("") -> (w8:string[][])  [unwired: 2 in]
          n9 = Spreadsheet String To Array(format string="%s", spreadsheet string=w9, array type (2D Dbl)=w8) -> (array=w1:string[][])  [unwired: 1 in]
          "Params list" <- w1
          n10 = for {
            tunnel: w1 -> [w15] mode=indexing
            tunnel: w4 -> [w18]
            tunnel: [w17] -> w3 mode=indexing
            n11 = Index Array(array=w15) -> (element #1=w14:string, element #2=w13:string)  [unwired: 2 in]
            n12 = Bundle By Name(cluster=w18, "Status"=w14, "Name"=w13, "Value"=0.0) -> (w17:T4)
          }
          n13 = local write "Default Parameters"(w3) -> ()
        }
        frame #1 {
          w22 = FALSE ("Open parameter editor")
          # "Edit # is a state variable telling the VI that the user asked to edit parameters or a macro."
          n14 = Index Array(array="Actions") -> (element=w27:T2)  [unwired: 1 in]
          n15 = Bundle(cluster=w27, "Toggle"=TRUE, "Open parameter editor"=w22, "Open MacroEditor"=w22, "Macro path"=path "", "Duration (s)"=0.001 ("Time to wait for parameters to change (s)"), "Parameters"="Default Parameters", "Comment"="") -> (→"Default Action":T2)  [unwired: 1 in]
          n16 = local write "Edit #"(i64 -1 ("Edit #")) -> ()
        }
      }
    }
    frame #1 {
      # "Run"
      n17 = while {
        stop <- "stop" stop-if-true
        n18 = event shown="[0] Timeout" {
          selector: _ -> [_ _ _ _ _ _]
          dyn-events: _ -> [_ _ _ _ _ _]
          timeout: 100 -> [_ _ _ _ _ _]
          event Timeout {
            n19 = event-data() -> ()  [unwired: 1 in, 3 out]
            n20 = stacked-sequence {
              seq-local: [_ _ _ w144 _ _] -> [_ _ _ _ w156 _]
              frame #0 {
                # "Check whether user has requested the parameter editor"
                n21 = local read "Edit #"() -> (w32:i32)
                n22 = Greater Or Equal To 0?(x=w32) -> (x >= 0?=w31:bool)
                n23 = case shown="True" w31 {
                  tunnel: w32 -> [_ w40]
                  frame False {
                    # "No request. Check again..."
                    n24 = local read "Actions"() -> (w37:T1)
                    n25 = for {
                      tunnel: w37 -> [w39] mode=indexing
                      tunnel: [w38] -> w36 mode=indexing
                      n26 = Unbundle By Name(w39) -> ("Open parameter editor"=w38:bool)
                    }
                    n27 = Boolean To (0,1)(Boolean=w36) -> (0, 1=w34:i16[])
                    n28 = Search 1D Array(1D array=w34, element=1) -> (index of element=→"Edit #":i32)  [unwired: 1 in]
                  }
                  frame True {
                    # "Editor requested."
                    n29 = stacked-sequence {
                      tunnel: w40 -> [w41 w80 _]
                      frame #0 {
                        # "Open editor and change parameters"
                        n30 = local read "Actions"() -> (w43:T1)
                        n31 = Index Array(array=w43, index=w41) -> (element=w44:T2)
                        n32 = Unbundle By Name(w44) -> ("Toggle"=w42:bool)
                        n33 = case shown="True" w42 {
                          tunnel: w41 -> [w45 w58]
                          frame False {
                            n34 = local read "Actions"() -> (w52:T1)
                            n35 = Index Array(array=w52, index=w45) -> (element=w51:T2)
                            n36 = Unbundle By Name(w51) -> ("Macro path"=w50:path)
                            n37 = Path To String(path=w50) -> (string=w49:string)
                            n38 = String Length(string=w49) -> (length=w48:i32)
                            n39 = Greater?(x=w48, y=1) -> (0:w47:bool)
                            n40 = case shown="True" w47 {
                              tunnel: w50 -> [_ w56]
                              frame False {
                                n41 = One Button Dialog(message="Not a good macro path", button name ("OK")="oops") -> ()  [unwired: 1 out]
                              }
                              frame True {
                                n42 = local read "System"() -> (w55:u16)
                                n43 = call "MacroEditor.vi"("System"=w55, "Save/Open Path"=w56, "Sub-vi'd (open)"=TRUE) -> ()  [unwired: 1 in, 1 out]
                              }
                            }
                          }
                          frame True {
                            n44 = case shown="0" w58 {
                              selector: w58 -> [w59 w68]
                              frame 0 {
                                # "0th element must refer to something, so use Default"
                                n45 = local read "Actions"() -> (w64:T1)
                                n46 = Index Array(array=w64, index=w59) -> (element=w63:T2)
                                n47 = local read "Default Parameters"() -> (w61:T3)
                                n48 = Unbundle By Name(w63) -> ("Parameters"=w62:T3)
                                n49 = call "ParameterEditor_new.vi"("Previous Parameters"=w61, "New Parameters"=w62) -> ("Output parameters"=w60:T3)
                                n50 = Bundle By Name(cluster=w63, "Parameters"=w60) -> (w65:T2)
                                n51 = local read "Edit #"() -> (w66:i32)
                                n52 = Replace Array Subset(array=w64, new element=w65, index=w66) -> (w67:T1)
                                n53 = local write "Actions"(w67) -> ()
                              }
                              frame Default {
                                # "Not 0th line: use previous line as reference"
                                n54 = local read "Actions"() -> (w75:T1)
                                n55 = Decrement(x=w68) -> (x-1=w73:i32)
                                n56 = Index Array(array=w75, index #1=w68, index #2=w73) -> (element #1=w72:T2, element #2=w74:T2)
                                n57 = Unbundle By Name(w74) -> ("Parameters"=w70:T3)
                                n58 = Unbundle By Name(w72) -> ("Parameters"=w71:T3)
                                n59 = call "ParameterEditor_new.vi"("Previous Parameters"=w70, "New Parameters"=w71) -> ("Output parameters"=w69:T3)
                                n60 = Bundle By Name(cluster=w72, "Parameters"=w69) -> (w76:T2)
                                n61 = local read "Edit #"() -> (w77:i32)
                                n62 = Replace Array Subset(array=w75, new element=w76, index=w77) -> (w78:T1)
                                n63 = local write "Actions"(w78) -> ()
                              }
                            }
                          }
                        }
                      }
                      frame #1 {
                        # "Restore 'No Request' state"
                        n64 = local read "Actions"() -> (w83:T1)
                        n65 = Index Array(array=w83, index=w80) -> (element=w84:T2)
                        n66 = Bundle By Name(cluster=w84, "Open parameter editor"=FALSE) -> (w82:T2)
                        n67 = Replace Array Subset(array=w83, new element=w82, index=w80) -> (w81:T1)
                        n68 = local write "Actions"(w81) -> ()
                        n69 = local write "Edit #"(-1 ("Edit #")) -> ()
                      }
                      frame #2 {
                        # "Propagate changes:\nAll 'unchanged' parameters inherit from the previous line (except on line 0)"
                        n70 = local read "Actions"() -> (w86:T1)
                        n71 = for {
                          tunnel: w86 -> [_] mode=indexing
                          i -> [w87]
                          n72 = local read "Actions"() -> (w88:T1)
                          n73 = case shown="Default" w87 {
                            tunnel: w88 -> [_ w97]
                            tunnel: w87 -> [_ w93]
                            frame 0 {
                            }
                            frame Default {
                              n74 = Decrement(x=w93) -> (x-1=w94:i32)
                              n75 = Index Array(array=w97, index #1=w93, index #2=w94) -> (element #1=w89:T2, element #2=w95:T2)
                              n76 = Unbundle By Name(w95) -> ("Parameters"=w91:T3)
                              n77 = Unbundle By Name(w89) -> ("Parameters"=w92:T3)
                              n78 = call "ParameterEditor_background_new.vi"("Previous Parameters"=w91, "New Parameters"=w92) -> ("Output parameters"=w90:T3)
                              n79 = Bundle By Name(cluster=w89, "Parameters"=w90) -> (w96:T2)
                              n80 = local read "Actions"() -> (w99:T1)
                              n81 = Replace Array Subset(array=w99, new element=w96, index=w93) -> (w98:T1)
                              n82 = local write "Actions"(w98) -> ()
                            }
                          }
                        }
                      }
                    }
                  }
                }
              }
              frame #1 {
                # "If number of lines has changed (added or removed elements), repropagate parameter changes"
                n83 = local read "Last Value"() -> (w102:i32)
                n84 = local read "Actions"() -> (w103:T1)
                n85 = Array Size(array=w103) -> (size(s)=w100:i32)
                n86 = Not Equal?(x=w100, y=w102) -> (x != y?=w101:bool)
                n87 = case shown="True" w101 {
                  tunnel: w103 -> [_ w105]
                  tunnel: w100 -> [_ w104]
                  frame False {
                    # "# lines hasn't changed"
                  }
                  frame True {
                    n88 = for {
                      tunnel: w105 -> [_] mode=indexing
                      i -> [w106]
                      n89 = local read "Actions"() -> (w107:T1)
                      n90 = case shown="Default" w106 {
                        tunnel: w107 -> [_ w110]
                        tunnel: w106 -> [_ w111]
                        frame 0 {
                          # "If a new line 0 was inserted, there could be trouble."
                        }
                        frame Default {
                          # "Not element 0. Good."
                          n91 = Decrement(x=w111) -> (x-1=w115:i32)
                          n92 = Index Array(array=w110, index #1=w111, index #2=w115) -> (element #1=w108:T2, element #2=w114:T2)
                          n93 = Unbundle By Name(w114) -> ("Parameters"=w117:T3)
                          n94 = Unbundle By Name(w108) -> ("Parameters"=w116:T3)
                          n95 = call "ParameterEditor_background_new.vi"("Previous Parameters"=w117, "New Parameters"=w116) -> ("Output parameters"=w118:T3)
                          n96 = Bundle By Name(cluster=w108, "Parameters"=w118) -> (w113:T2)
                          n97 = local read "Actions"() -> (w112:T1)
                          n98 = Replace Array Subset(array=w112, new element=w113, index=w111) -> (w109:T1)
                          n99 = local write "Actions"(w109) -> ()
                        }
                      }
                    }
                    "Last Value" <- w104
                  }
                }
              }
              frame #2 {
                # "If a macro is in the path and the action type is macro, \nupdate comments and duration from macro"
                n100 = local read "LastMods"() -> (w120:timestamp[])
                n101 = local read "Actions"() -> (w122:T1)
                n102 = for {
                  tunnel: w122 -> [w127] mode=indexing
                  tunnel: [w126] -> w119 mode=indexing
                  tunnel: w120 -> [w136]
                  tunnel: [w125] -> w121 mode=indexing
                  i -> [w135]
                  n103 = Unbundle By Name(w127) -> ("Macro path"=w129:path, "Toggle"=w130:bool)
                  n104 = Index Array(array=w136, index=w135) -> (element=w128:timestamp)
                  n105 = Not(x=w130) -> (.not. x?=w131:bool)
                  n106 = File/Directory Info(path=w129) -> (last mod=w125:timestamp, error out=w123:errorcluster)  [unwired: 1 in, 5 out]
                  n107 = Not Equal?(x=path "", y=w129) -> (x != y?=w132:bool)
                  n108 = call <vilib>:"Clear Errors.vi"("error in (no error)"=w123) -> ()  [unwired: 5 in, 2 out]
                  n109 = Not Equal?(x=w125, y=w128) -> (x != y?=w124:bool)
                  n110 = Compound Arithmetic op=AND(w132, w131, w124) -> (w133:bool)
                  n111 = case shown="True" w133 {
                    tunnel: w129 -> [_ w143]
                    tunnel: w127 -> [w137 w141]
                    tunnel: [w137 w139] -> w126
                    frame False {
                    }
                    frame True {
                      n112 = call "XMLtoMacro.vi"("XML File Path"=w143) -> ("MacroSaveCluster"=w142:T5)
                      n113 = Unbundle By Name(w142) -> ("Macro Description"=w140:string, "Total Time (s)"=w138:dbl)
                      n114 = Bundle By Name(cluster=w141, "Comment"=w140, "Duration (s)"=w138) -> (w139:T2)
                    }
                  }
                }
                "LastMods" <- w121
                n115 = local write "Actions"(w119) -> ()
              }
              frame #3 {
                # "Update total time and # actions"
                n116 = local read "Actions"() -> (w146:T1)
                n117 = for {
                  tunnel: w146 -> [w155] mode=indexing
                  tunnel: [w150] -> w144 mode=indexing
                  n118 = Unbundle By Name(w155) -> ("Duration (s)"=w151:dbl, "Toggle"=w152:bool, "Reps"=w148:i32)
                  n119 = Add(x="Param Buffer (200 ms)", y=w151) -> (x+y=w153:dbl)
                  n120 = Select(t=w153, s=w152, f=w151) -> (s? t:f=w149:dbl)
                  n121 = Multiply(x=w149, y=w148) -> (x*y=w150:dbl)
                }
                n122 = Array Size(array=w146) -> (size(s)=→"# Actions":i32)
                n123 = Add Array Elements(numeric array=w144) -> (sum=→"Total Time (s)":dbl)
              }
              frame #4 {
                # "update sidebar"
                n124 = flat-sequence {
                  tunnel: w156 -> [w159]
                  frame #0 {
                    n125 = for {
                      tunnel: w159 -> [w161] mode=indexing
                      tunnel: [w163] -> w158 mode=indexing
                      shift-right: [w162] -> _
                      shift-left: 0.0 -> [w160]
                      i -> [w164]
                      n126 = Add(x=w161, y=w160) -> (x+y=w162:dbl)
                      n127 = Bundle(w164, w160) -> (w163:cluster{i32, dbl})  [unwired: 1 in]
                    }
                    "InfoArray" <- w158
                  }
                  frame #1 {
                    n128 = property on="Actions" class="Arr (strict)"() -> ("Index Values"=w165:u32[])  [unwired: 2 in, 2 out]
                    n129 = property on="InfoArray" class="Arr (strict)"("Index Values"=w165) -> ()  [unwired: 2 in, 2 out]
                  }
                }
              }
              frame #5 {
                # "wait 100 ms; I think this helps to keep the QEditor from overwriting values that the user enters manually"
                n130 = Wait (ms)(milliseconds to wait=100) -> ()  [unwired: 1 out]
              }
            }
          }
          event "New": Value Change {
            # "Scroll back up to the top"
            n131 = event-data() -> ()  [unwired: 1 in, 5 out]
            n132 = local read "Default Action"() -> (w169:T2)
            n133 = property on="Actions" class="Arr (strict)"("Index Values"=u32[] [0]) -> ()  [unwired: 2 in, 2 out]
            n134 = local write "Save"(FALSE) -> ()
            n135 = Initialize Array(w169, 1 ("dimension size")) -> (w170:T2[])
            n136 = local write "Actions"(w170) -> ()
          }
          event "Save": Value Change {
            n137 = event-data() -> ()  [unwired: 1 in, 3 out]
            n138 = stacked-sequence {
              seq-local: [w173 _] -> [_ w195]
              seq-local: [w172 _] -> [_ w194]
              frame #0 {
                # "Check for empty paths"
                n139 = local read "Actions"() -> (w175:T1)
                n140 = for {
                  tunnel: w175 -> [w181] mode=indexing
                  tunnel: [w178] -> w174 mode=indexing
                  tunnel: [w177] -> w172 mode=indexing if=w176
                  n141 = Unbundle By Name(w181) -> ("Toggle"=w180:bool, "Macro path"=w177:path)
                  n142 = case shown="False" w180 {
                    tunnel: w177 -> [w185 _]
                    tunnel: "Error: Empty path or no such macro file.\nFix this or else file will not be saved." ("message") -> [w188 _]
                    tunnel: [w183 TRUE ("Save")] -> w178
                    tunnel: [w182 FALSE ("file or folder exists?")] -> w176
                    frame False {
                      # "seems to\nneed this"
                      # "Macro"
                      n143 = call <vilib>:"Check if File or Folder Exists.vi"("path"=w185) -> ("file or folder exists?"=w182:bool)  [unwired: 8 in, 2 out]
                      n144 = Not Equal?(x=w185, y=path "") -> (x != y?=w184:bool)
                      n145 = And(x=w182, y=w184) -> (x .and. y?=w186:bool)
                      n146 = case shown="True" w186 {
                        tunnel: w188 -> [w190 _]
                        tunnel: [w189 TRUE ("Save")] -> w183
                        frame False {
                          w189 = FALSE ("Save")
                          # "No such file"
                          n147 = One Button Dialog(message=w190) -> ()  [unwired: 1 in, 1 out]
                          n148 = local write "Save"(w189) -> ()
                        }
                        frame True {
                          # "OK"
                        }
                      }
                    }
                    frame True {
                    }
                  }
                }
                n149 = And Array Elements(Boolean array=w174) -> (logical AND=w173:bool)
              }
              frame #1 {
                # "Only save if paths are good"
                n150 = case shown="True" w195 {
                  tunnel: w194 -> [_ w196]
                  frame False {
                  }
                  frame True {
                    # "Save cue, and copy all macros referenced by cue, for posterity"
                    n151 = stacked-sequence {
                      seq-local: [_ w203 _] -> [_ _ w212]
                      seq-local: ["Save/Open Path" _ _] -> [_ w202 _]
                      tunnel: w196 -> [_ _ w213]
                      frame #0 {
                        # "Save Cue"
                        n152 = local read "Total Time (s)"() -> (w199:dbl)
                        n153 = local read "Actions"() -> (w198:T1)
                        n154 = Bundle("Total Time (s)"=w199, "Cue Description"="Cue Description") -> (w201:T8)  [unwired: 1 in]
                        n155 = call "QtoXML.vi"("output cluster"=w201, "Actions"=w198, "XML File Path"="Save/Open Path") -> ()  [unwired: 1 in]
                      }
                      frame #1 {
                        # "Make folder in same place as the cue"
                        n156 = Strip Path(path=w202) -> (stripped path=w207:path)  [unwired: 1 out]
                        n157 = call <vilib>:"Get File Extension.vi"("file"=w202) -> ("filename without extension"=w208:string)  [unwired: 6 in, 4 out]
                        n158 = Build Path(base path=w207, name or relative path=w208) -> (appended path=w206:path)
                        n159 = call <vilib>:"Check if File or Folder Exists.vi"("path"=w206) -> ("file or folder exists?"=w205:bool, "dup path"=w204:path)  [unwired: 8 in, 1 out]
                        n160 = case shown="True" w205 {
                          tunnel: w204 -> [w210 w211]
                          tunnel: [w209 w211] -> w203
                          frame False {
                            n161 = Create Folder(path (use dialog)=w210) -> (created path=w209:path)  [unwired: 2 in, 2 out]
                          }
                          frame True {
                          }
                        }
                      }
                      frame #2 {
                        # "Copy macros to that folder"
                        n162 = for {
                          tunnel: w213 -> [w215] mode=indexing
                          tunnel: w212 -> [w214]
                          n163 = Strip Path(path=w215) -> (name=w216:string)  [unwired: 1 out]
                          n164 = Build Path(base path=w214, name or relative path=w216) -> (appended path=w218:path)
                          n165 = Copy(9:TRUE ("overwrite (F)"), 10:w218, 11:w215) -> ()  [unwired: 2 in, 3 out]
                        }
                      }
                    }
                  }
                }
              }
            }
          }
          event "Open": Value Change {
            n166 = event-data() -> ()  [unwired: 1 in, 3 out]
            n167 = local read "Save/Open Path"() -> (w219:path)
            n168 = call <vilib>:"Check if File or Folder Exists.vi"("path"=w219) -> ("file or folder exists?"=w220:bool)  [unwired: 8 in, 2 out]
            n169 = local write "Save"(FALSE) -> ()
            n170 = case shown="True" w220 {
              tunnel: w219 -> [_ w227]
              frame False {
                n171 = One Button Dialog(message="Can't open file because it doesn't exist") -> ()  [unwired: 1 in, 1 out]
              }
              frame True {
                n172 = call "XMLtoQ.vi"("XML File Path"=w227) -> ("Cue out"=w223:T1, "Description"=w226:T9)
                n173 = Unbundle(w226) -> ("Total\nTime (s)"=w225:dbl, "Cue Description"=w224:string)
                n174 = local write "Actions"(w223) -> ()
                n175 = local write "Cue Description"(w224) -> ()
                n176 = local write "Total Time (s)"(w225) -> ()
              }
            }
          }
          event "Cue Description": Mouse Down {
            # "(stale)"
            n177 = event-data() -> ()  [unwired: 1 in, 8 out]
            n178 = local write "Save"(FALSE ("Save")) -> ()
          }
          event "Add macros": Value Change {
            # "(stale)"
            n179 = event-data() -> ()  [unwired: 1 in, 6 out]
            n180 = Strip Path(path="First file") -> (stripped path=w229:path)  [unwired: 1 out]
            n181 = local write "Save"(FALSE ("Save")) -> ()
            n182 = call <vilib>:"Recursive File List.vi"("pattern"="*US*.mac", "Folder Path"=w229) -> ("All Files in Dir"=w232:path[])  [unwired: 5 in, 4 out]
            n183 = call <vilib>:"Recursive File List.vi"("pattern"="*DS*.mac", "Folder Path"=w229) -> ("All Files in Dir"=w239:path[])  [unwired: 5 in, 4 out]
            n184 = for {
              tunnel: w239 -> [w250] mode=indexing
              tunnel: "First file" -> [w253]
              tunnel: "Last file" -> [w252]
              tunnel: [w250] -> w237 mode=indexing if=w245
              tunnel: w232 -> [w246] mode=indexing
              tunnel: [w246] -> w231 mode=indexing if=w245
              n185 = Greater Or Equal?(x=w250, y=w253) -> (x >= y?=w248:bool)
              n186 = Less Or Equal?(x=w250, y=w252) -> (x <= y?=w251:bool)
              n187 = And(x=w248, y=w251) -> (x .and. y?=w249:bool)
              n188 = Select(t=w248, s="To end", f=w249) -> (s? t:f=w245:bool)
            }
            n189 = local read "Actions"() -> (w242:T1)
            n190 = Index Array(array=w242) -> (element=w243:T2)  [unwired: 1 in]
            n191 = for {
              tunnel: w243 -> [w266]
              shift-right: [w264] -> w236
              shift-left: w242 -> [w267]
              tunnel: "Insert at Action" -> [w262]
              tunnel: w237 -> [w257] mode=indexing
              tunnel: "Replace" -> [w260]
              tunnel: w231 -> [w258] mode=indexing
              tunnel: "US+DS" -> [w256]
              i -> [w259]
              n192 = case shown="False" w256 {
                tunnel: w259 -> [_ w272]
                tunnel: ["US/DS" w269] -> w255
                frame False {
                }
                frame True {
                  n193 = Quotient & Remainder(x=w272, y=2) -> (x-y*floor(x/y)=w270:i32)  [unwired: 1 out]
                  n194 = Equal To 0?(x=w270) -> (x = 0?=w269:bool)
                }
              }
              n195 = Select(t=w258, s=w255, f=w257) -> (s? t:f=w254:path)
              n196 = Bundle By Name(cluster=w266, "Toggle"=FALSE, "Macro path"=w254) -> (w263:T2)
              n197 = Add(x=w259, y=w262) -> (x+y=w261:i32)
              n198 = case shown="True" w260 {
                tunnel: w267 -> [w276 w278]
                tunnel: [w275 w277] -> w264
                tunnel: w263 -> [w274 w279]
                tunnel: w261 -> [w273 w280]
                frame False {
                  n199 = Insert Into Array(array=w276, index=w273, new element=w274) -> (w275:T1)
                }
                frame True {
                  n200 = Replace Array Subset(array=w278, new element=w279, index=w280) -> (w277:T1)
                }
              }
            }
            n201 = local write "Actions"(w236) -> ()
          }
        }
      }
    }
  }
